vi "slow_control_2_17.vi"() -> ()   [LabVIEW 2018]
uses:
  4623b864-5764-45c6-9cb2-3e18237880ca.vi
  fa57f61f-0bb9-49ac-92eb-fcb40add4dbb.vi
  <vilib>/DAQmx/read.llb/DAQmx Read (Analog 1D DBL NChan 1Samp).vi
  ffb0d1b3-ef19-4e2e-b36e-7277177ef4b3.vi
  9a1acc8a-69db-4048-9e4c-bb07d66d2422.vi
  <vilib>/DAQmx/create/channels.llb/DAQmx Create Channel (AI-Voltage-Basic).vi
  <vilib>/DAQmx/create/channels.llb/DAQmx Create Channel (AI-Current-Basic).vi
  <vilib>/DAQmx/create/channels.llb/DAQmx Create Channel (AI-Temperature-RTD).vi
  <vilib>/DAQmx/miscellaneous.llb/DAQmx Fill In Error Info.vi
  <vilib>/Utility/file.llb/Read Delimited Spreadsheet (string).vi
  <instrlib>/Lake Shore 335/Lake Shore 335.lvlib
  <instrlib>/CAEN PSM/CAEN PSM.lvlib
  <resource>/objmgr/daqmx.rc
panel:
  out "Setpoint (°C)":dbl
  out "Heater Range":i32
  out "Heater (°C)":dbl
  out "Coldhead (°C)":dbl
  out "Cycle number":i32
  out "Alarm state":bool
  out "Timestamp last \nmeasured (UPS)":timestamp
  out "Auto-clear":bool
  in  "Auto-clear data?":bool
  in  "Clear data":bool
  in  "Clear data every N cycles":dbl=1000000.0
  in  "N samples":i32=30
  out "Average Flow (SLPM)":dbl caption="Flow (SLPM)"
  out "CAEN Ch. Names":string[](array[string])
  in  "Cycles to execute":dbl=5.0 format="%#_13g"
  out "Detector Pressure":dbl
  in  "N samples":i32=20
  in  "Allows tabs on \nfront panel":T1(tab)
  in  "Anode ch.":enum16{"1", "2", "3", "4"}(ring)=enum."3"
  in  "CAEN unit selector":enum16{"CAEN 1", "CAEN 2"}(ring)
  in  "Multipliers":dbl[](array[numeric])=[1.0, 1.0, 1.0, 1.0, 1.0, 1.0, 1.0, 1.0]
  in  "Offsets\nsubtracted":dbl[](array[numeric])=[0.0, 0.0, 0.0, 0.0, 0.0, 0.0, 0.0, 0.0]
  in  "Channel Names (9207, ai8:15)":string[](array[string])=["i0", "i1", "i2", "i3", "i4", "i5", "i6", "i7"] caption="\"Other\""
  in  "Flow meter input:":u16(ring)=3 items=["v0", "v1", "v2", "v3", "v4", "v5", "v6", "v7"]
  in  "Detector pressure input:":u16(ring) items=["v0", "v1", "v2", "v3", "v4", "v5", "v6", "v7"]
  in  "Channel Names (9207, ai0:7)":string[](array[string])=["v0", "v1", "v2", "v3", "v4", "v5", "v6", "v7"] caption="\"Other\""
  in  "Multipliers":dbl[](array[numeric])=[1.0, 1.0, 1.0, 1.0, 1.0, 1.0, 1.0, 1.0]
  in  "Offsets\nsubtracted":dbl[](array[numeric])=[0.0, 0.0, 0.0, 0.0, 0.0, 0.0, 0.0, 0.0]
  in  "Voltage channels":tag[](array[tag])=["9207/ai0", "9207/ai1", "9207/ai2", "9207/ai3", "9207/ai4", "9207/ai5", "9207/ai6", "9207/ai7"]
  in  "COM-ports CAEN":refnum<visa-resource-name>[](array[refnum])
  in  "ID Query":bool
  in  "COM-port LakeShore":refnum<visa-resource-name>
  in  "PID settings":cluster{"P":dbl, "I":dbl, "D":dbl}={"P"=50.0, "I"=20.0, "D"=120.0}
  in  "Current channels":tag[](array[tag])=["9207/ai8", "9207/ai9", "9207/ai10", "9207/ai11", "9207/ai12", "9207/ai13", "9207/ai14", "9207/ai15"]
  in  "Channel Names (CAEN)":string[](array[string])=["PMT 1", "PMT 2", "Anode", "Cathode", "Top gate", "Bottom gate", "Other 1", "Other 2"]
  in  "RTD Type":i32(ring)=10071 items=["Pt3750"=12481, "Pt3851"=10071, "Pt3911"=12482, "Pt3916"=10069, "Pt3920"=10053, "Pt3928"=12483, "Custom"=10137]
  in  "Module 1 channels (slot 1)":tag[](array[tag])=["cDAQ2Mod2/ai0", "cDAQ2Mod2/ai1", "cDAQ2Mod2/ai2", "cDAQ2Mod2/ai3", "cDAQ2Mod2/ai4", "cDAQ2Mod2/ai5", "cDAQ2Mod2/ai6", "cDAQ2Mod2/ai7"]
  in  "Resistance Configuration":i32(ring)=3 items=["3-Wire"=3, "4-Wire"=4]
  in  "R (T = 0°C):":dbl=100.0 format="%_4g"
  in  "B":dbl
  in  "A":dbl
  in  "C":dbl
  in  "Module 2 channels (slot 2)":tag[](array[tag])=["cDAQ2Mod3/ai0", "cDAQ2Mod3/ai1", "cDAQ2Mod3/ai2", "cDAQ2Mod3/ai3", "cDAQ2Mod3/ai4", "cDAQ2Mod3/ai5", "cDAQ2Mod3/ai6", "cDAQ2Mod3/ai7"]
  in  "Shut off heater \nif Alarm is active":bool=TRUE
  in  "Re-save headers":bool
  in  "Resistance Configuration":i32(ring)=3 items=["3-Wire"=3, "4-Wire"=4]
  in  "Module 3 channels":tag[](array[tag])
  in  "RTD Type":i32(ring)=12481 items=["Pt3750"=12481, "Pt3851"=10071, "Pt3911"=12482, "Pt3916"=10069, "Pt3920"=10053, "Pt3928"=12483, "Custom"=10137]
  in  "R (T = 0°C)":dbl=1000.0 format="%0.1f"
  in  "Ignore Initialization Errors":bool=TRUE caption="Ignore init. errors?"
  out "Started up?":bool
  in  "9216 Timing Mode":i32(ring)=14712 items=["High Resolution"=10195, "High Speed"=14712]
  in  "9207 Timing Mode":i32(ring)=14712 items=["High Resolution"=10195, "High Speed"=14712]
  in  "9226 Timing Mode":i32(ring)=14712 items=["High Resolution"=10195, "High Speed"=14712]
  in  "Kill all channels (Trip)":bool
  in  "Scale.Range:Minimum 8":dbl
  in  "Scale.Range:Maximum 8":dbl=4000.0
  in  "Scale.Range:Minimum 7":dbl
  in  "Scale.Range:Maximum 7":dbl=4000.0
  in  "Scale.Range:Minimum 6":dbl=-3000.0
  in  "Scale.Range:Maximum 6":dbl
  in  "Scale.Range:Minimum 5":dbl
  in  "Scale.Range:Maximum 5":dbl=3000.0
  in  "Scale.Range:Minimum 4":dbl=-5000.0
  in  "Scale.Range:Maximum 4":dbl
  in  "Scale.Range:Maximum 3":dbl=4000.0
  in  "Scale.Range:Minimum 3":dbl
  in  "Scale.Range:Maximum 2":dbl=1000.0
  in  "Scale.Range:Minimum 2":dbl
  out "CAEN 1.1":dbl(knob) scale=0.0..1000.0
  out "CAEN 1.1":string
  in  "Scale.Range:Maximum":dbl=1000.0
  in  "Scale.Range:Minimum":dbl
  out "CAEN 2.3 2":string
  out "CAEN 2.2 2":string
  out "Channel Names":string[](array[string])
  out "CAEN 2.3":dbl(knob) scale=0.0..4000.0
  out "CAEN 2.2":dbl(knob) scale=0.0..4000.0
  out "CAEN 2.1":string
  out "CAEN 2.0":string
  out "CAEN 1.3":string
  out "CAEN 1.2":string
  out "CAEN 1.0":string
  out "Channel Names":string[](array[string])
  in  "Set to zero (ramp down)":bool
  out "CAEN 2.1":dbl(knob) scale=0.0..-3000.0
  out "CAEN 2.0":dbl(knob) scale=0.0..3000.0
  in  "Apply Voltage":bool
  in  "VSet (V)":dbl[](array[numeric])
  in  "IMax (uA)":sgl[](array[numeric])
  in  "VMax (V)":u16[](array[numeric])
  out "CAEN 1.3":dbl(knob) scale=0.0..-5000.0
  out "CAEN 1.2":dbl(knob) scale=0.0..4000.0
  out "CAEN 1.0":dbl(knob) scale=0.0..1000.0
  out "Vmon (V)":dbl[](array[numeric])
  out "IMon (uA)":dbl[](array[numeric])
  in  "Reset anode\nperiodically?":bool
  in  "Kill every Y minutes":i32=10
  in  "Keep off for X seconds":i32=10
  out "?":bool
  out "Killed":bool
  out "Restarted":bool
  out "Anode timers":timestamp[](array[timestamp])
  out "Seconds until \nanode autokill":dbl format="%.2g"
  out "Seconds until \nanode reset":dbl format="%.2g"
  in  "Temperature channel selector":u16(ring) items=["0"=0, "1"=1, "2"=2, "3"=3, "4"=4, "5"=5, "6"=6, "7"=7, "Average"=666]
  out "Heater power (%)":cluster{timestamp[], dbl[]}[](graph)
  out "Flow (SLPM)":cluster{timestamp[], dbl[]}[](graph)
  out "9207 (ai 0:7, Volts)":cluster{timestamp[], dbl[]}[](graph)
  out "Phase Diagram":cluster{"X":dbl, "Y":dbl}[](graph)
  out "Setup Temperature (9216 0:15, °C)":cluster{timestamp[], dbl[]}[](graph)
  out "LakeShore readings":dbl[](array[numeric])
  out "Low Temperature (9226 0:7 and LakeShore A;B, °C)":cluster{timestamp[], dbl[]}[](graph)
  in  "Reset?":bool
  out "Integrated Flow (SL)":dbl
  in  "Pause?":bool
  in  "Setpoint (°C)":dbl=-100.0 format="%.1f"
  in  "Heater range":u16(ring) items=["Off", "Low (On)", "Medium", "High"]
  out "element 2":bool
  out "element":bool
  in  "T 8":bool
  in  "T 7":bool
  out "Minimum input voltage measured":dbl
  out "NI mod 2&3 status":bool
  in  "NI mod 2&3":bool
  in  "NI mod 1":bool
  in  "CAEN 2":bool
  in  "CAEN 1":bool
  in  "LakeShore":bool
  out "Comm. status":bool
  out "LakeShore status":bool
  out "NI mod1 (P) status":bool
  out "CAEN 1 status":bool
  out "CAEN 2 status":bool
  out "Initialization status":bool
  in  "\"Sound\" alarm":bool
  in  "Sound alarm\nFrequency (Hz)":dbl=1260.0
  in  "Send status email now":bool
  out "Email error":i32
  out "source":string
  in  "Number of Bonus lines":i32=1
  out "Names (optional)":string[](array[string])
  in  "Send daily email?":bool=TRUE
  in  "Phone numbers":string[](array[string])
  out "Alarm (or test) message":string
  in  "Alarm\nMaster switch":bool
  in  "Repeat Alarm SMS\nevery N minutes":dbl=15.0
  in  "Test alarm":bool
  out "Warning":bool
  in  "UPS":bool
  in  "UPS Voltage \nLower Threshold":dbl=220.0
  out "Det. P. warning":bool
  out "Boolean 6":bool
  out "Boolean 5":bool
  out "Boolean 4":bool
  out "Boolean 3":bool
  out "Boolean 2":bool
  out "Boolean":bool
  in  "T 6":bool
  in  "T 5":bool
  in  "T 4":bool
  in  "T 3":bool
  in  "T 2":bool
  in  "T 1":bool
  in  "Detector Pressure:":bool
  in  "Overpressure threshold":dbl
  in  "Underpressure threshold":dbl
  in  "High Temp threshold":dbl format="%#_13g"
  in  "Low Temp threshold":dbl format="%#_13g"
  out "Alarm active 2":bool
  out "SMS error":string
  out "Status email preview":string
  in  "Send status email at time:":string="14:00"
  in  "Email Addresses":string[](array[string])
  in  "return address":string="xamsups@gmail.com"
  out "NI 9226":errorcluster
  in  "HV Channel status":string="Click the button to request the latest High Voltage channel status.\nView another channel with the arrows, or typing 0 through 3."
  out "CAEN 1":T2(array[cluster])
  out "CAEN 2":T2(array[cluster])
  in  "Query HV status":bool
  in  "LabVIEW error code":string="Google this"
  in  "String 7":string="A checkmark means \"No error\" and false. A red X means an error occurred"
  out "\"status\"":bool
  in  "\"source\"":string="This may show two things: the latest executed VI in the task chain, in reverse order, or: which VI produced an error, with a short description. If the error can't easily be resolved, google the code."
  out "NI 9216 x2":errorcluster
  out "CAEN 1":errorcluster
  out "CAEN 2":errorcluster
  out "Lakeshore":errorcluster
  out "NI 9207":errorcluster
  out "Temp A":dbl
  out "Temp B":dbl
  in  "Temperature Channel Selector":u16(ring) items=["0", "1", "2", "3", "4", "5", "6", "7"]
  out "Historical Large Phase Diagram":cluster{dbl[], dbl[]}[](graph)
  out "Large Phase Diagram":cluster{"X":dbl, "Y":dbl}[](graph)
  in  "Temperature Channel Selector":u16(ring) items=["0"=0, "1"=1, "2"=2, "3"=3, "4"=4, "5"=5, "6"=6, "7"=7, "Average"=666]
  out "PT1000 data":dbl[](array[numeric]) format="%0.2f"
  out "9207 (V; A) Converted":dbl[](array[numeric])
  out "9216 #1 (°C)":dbl[](array[numeric])
  out "9216 #2 (°C)":dbl[](array[numeric])
  out "Raw readouts (V, mA)":dbl[](array[numeric]) format="%0.2f"
  out "Det.P input #":i32
  out "Flow input #":i32
  out "PT100 data":dbl[](array[numeric]) format="%0.2f"
  out "Polarity signs":dbl[](array[numeric])
  out "9207 (ai 8:15, Amperes)":cluster{timestamp[], dbl[]}[](graph)
  in  "Kill voltage":bool
  in  "stop":bool
  out "Voltages":dbl[](array[numeric])
  out "Time until next cycle":dbl format="%.3g"
  in  "Time per cycle (s)":i32=2 caption="Time Target (s)"
  # "Moving Averages"
  # "CAEN settings"
  # "NI 9216 Temperature settings"
  # "NI 9207 Voltage settings"
  # "NI 9207 Current settings"
  # "If RTD type is custom,\nspecify the Callendar-\nVan Dusen parameters"
  # "Anode connected to:"
  # "Channel:"
  # "Lakeshore settings"
  # "NI 9226 Temperature settings"
  # "Miscellaneous"
  # "Gain (P) (XX.X)"
  # "Reset (I) (XX.X)"
  # "Rate (D) (X.X%)"
  # "Data"
  # "Scale:"
  # "to"
  # "to"
  # "Scale:"
  # "Time of last reset"
  # "Time of last reactivation"
  # "to"
  # "Scale:"
  # "to"
  # "Scale:"
  # "Settings"
  # "Scale:"
  # "to"
  # "Scale:"
  # "to"
  # "Scale:"
  # "to"
  # "to"
  # "Scale:"
  # "Alarm indicators and arms"
  # "Detector Thresholds"
  # "Daily status email"
  # "SMS and sound alarm"
  # "Arms\nUp = Active"
  # "Alarm arms and warning lights"
  # "Temperature channels:"
  # "Uninterruptable Power Supply"
  # "Task/error information"
  # "High Voltage channel status"
  # "Error info example"
  # "Channel"
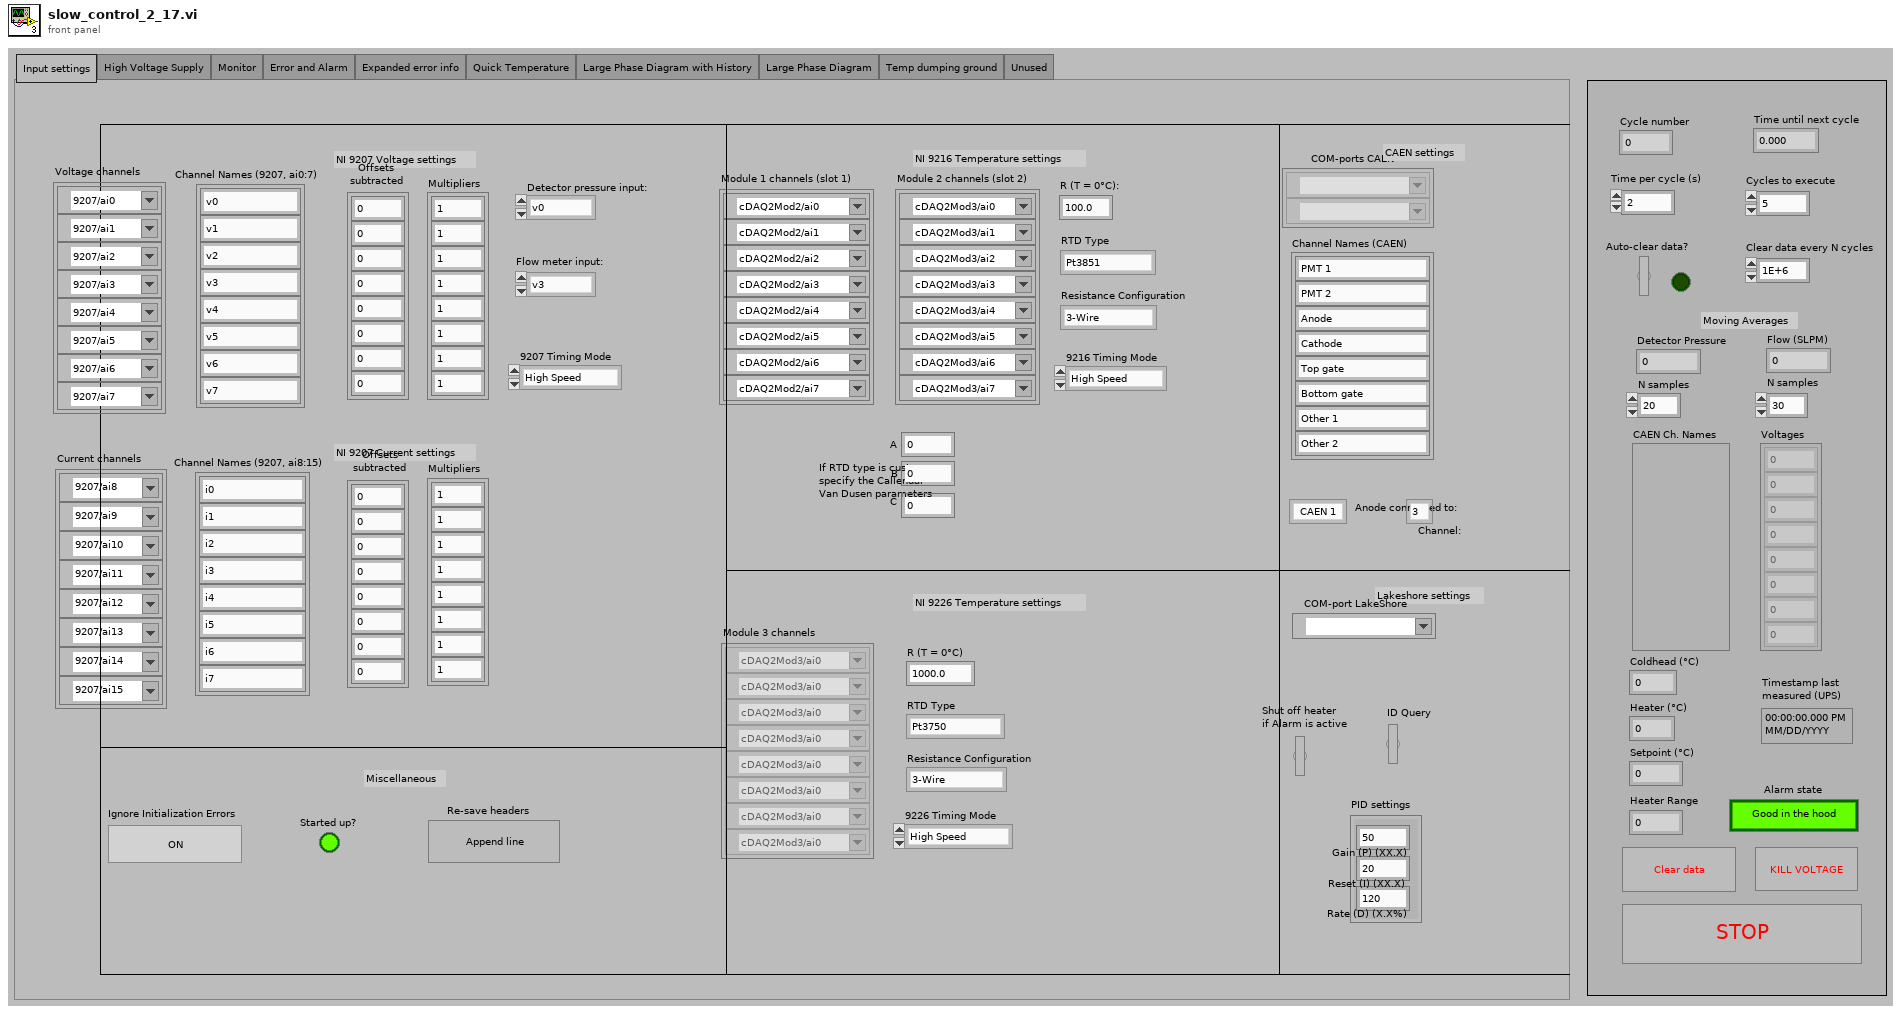
[diagram p1: front panel]
types:
  T1 = enum32{"Input settings", "High Voltage Supply", "Monitor", "Error and Alarm", "Expanded error info", "Quick Temperature", "Large Phase Diagram with History", "Large Phase Diagram", "Temp dumping ground", "Unused"}
  T2 = cluster{"ON":bool, "RUP":bool, "RDW":bool, "OVC":bool, "OVV":bool, "UNV":bool, "MAXV":bool, "TRIP":bool, "OVP":bool, "OVT":bool, "DIS":bool, "KILL":bool, "ILK":bool, "NOCAL":bool}[]
  T3 = cluster{"Baud Rate":u32, "Parity":u16, "Data Bits":u16, "Stop Bits":u16, "Flow Control":u16}
  T4 = typedef "CAEN PSM.lvlib/BoardHandle.ctl" = cluster{"VISA resource name":refnum<visa-resource-name>, "Board address":u8, "NChannels":u8}
  T5 = cluster{"task out":refnum<k21>, "error out":errorcluster}
  T6 = cluster{"VISA resource name out":refnum<visa-resource-name>, "error out":errorcluster}
  T7 = cluster{"VISA resource name":refnum<visa-resource-name>, "Board address":u8, "NChannels":u8}[]
  T8 = cluster{"VISA resource name":refnum<visa-resource-name>, "Board address":u8, "NChannels":u8}
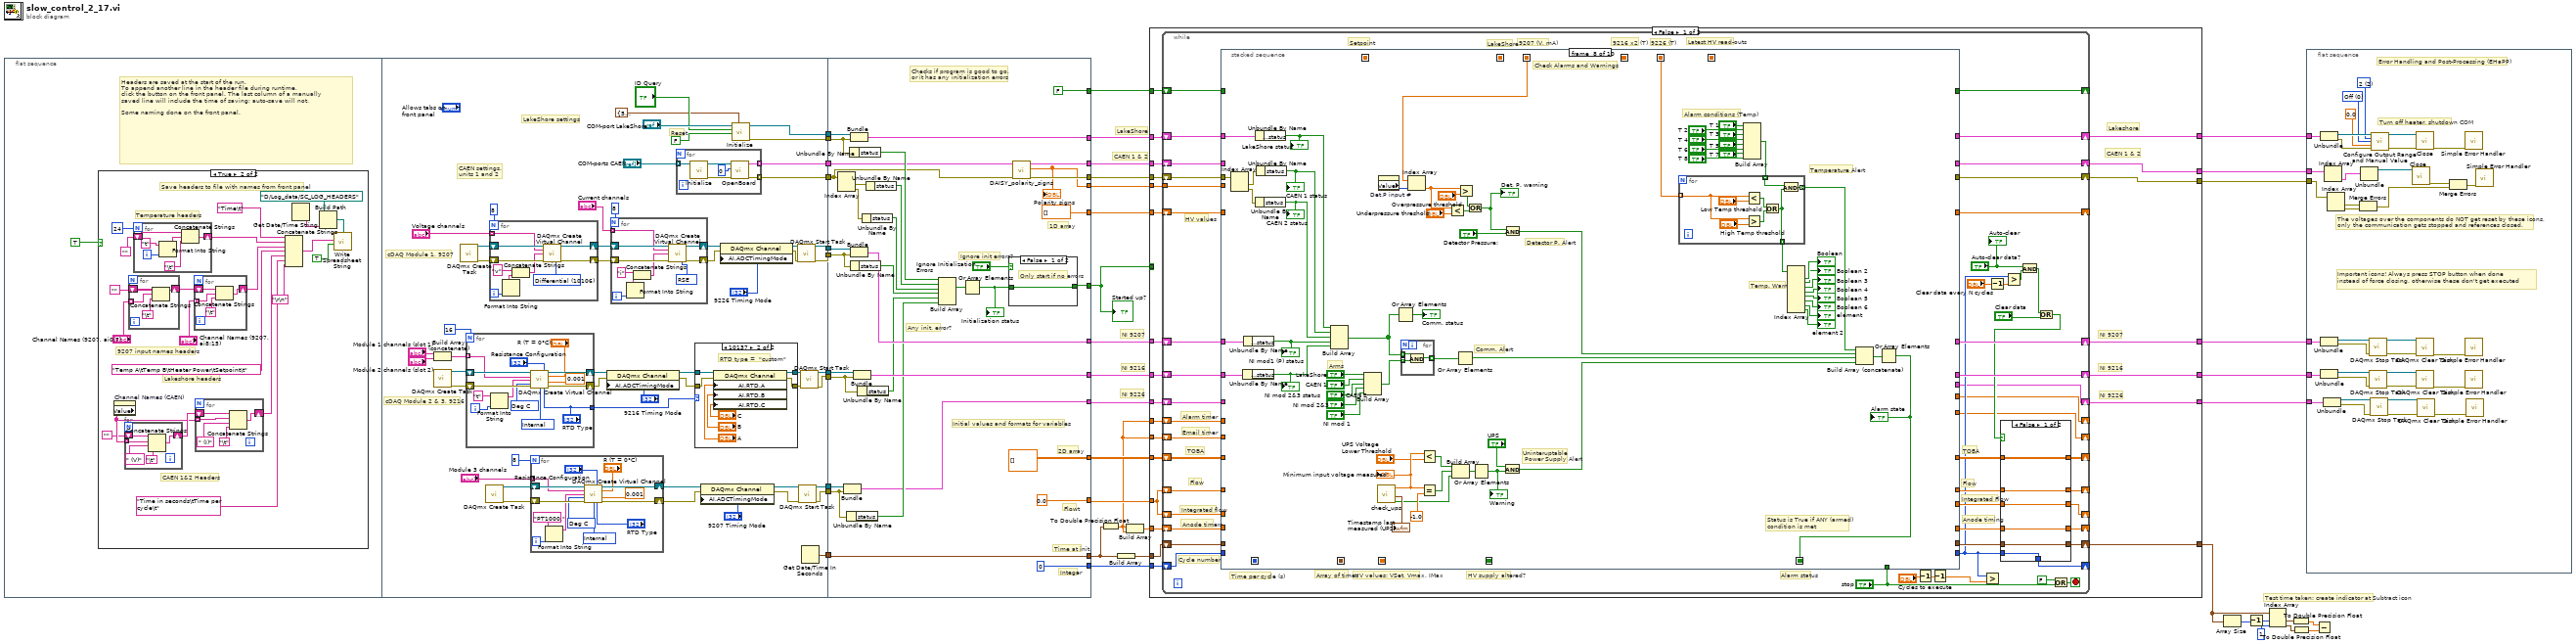
[diagram p0: block diagram]
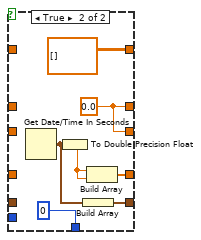
[diagram p2: hidden frame]
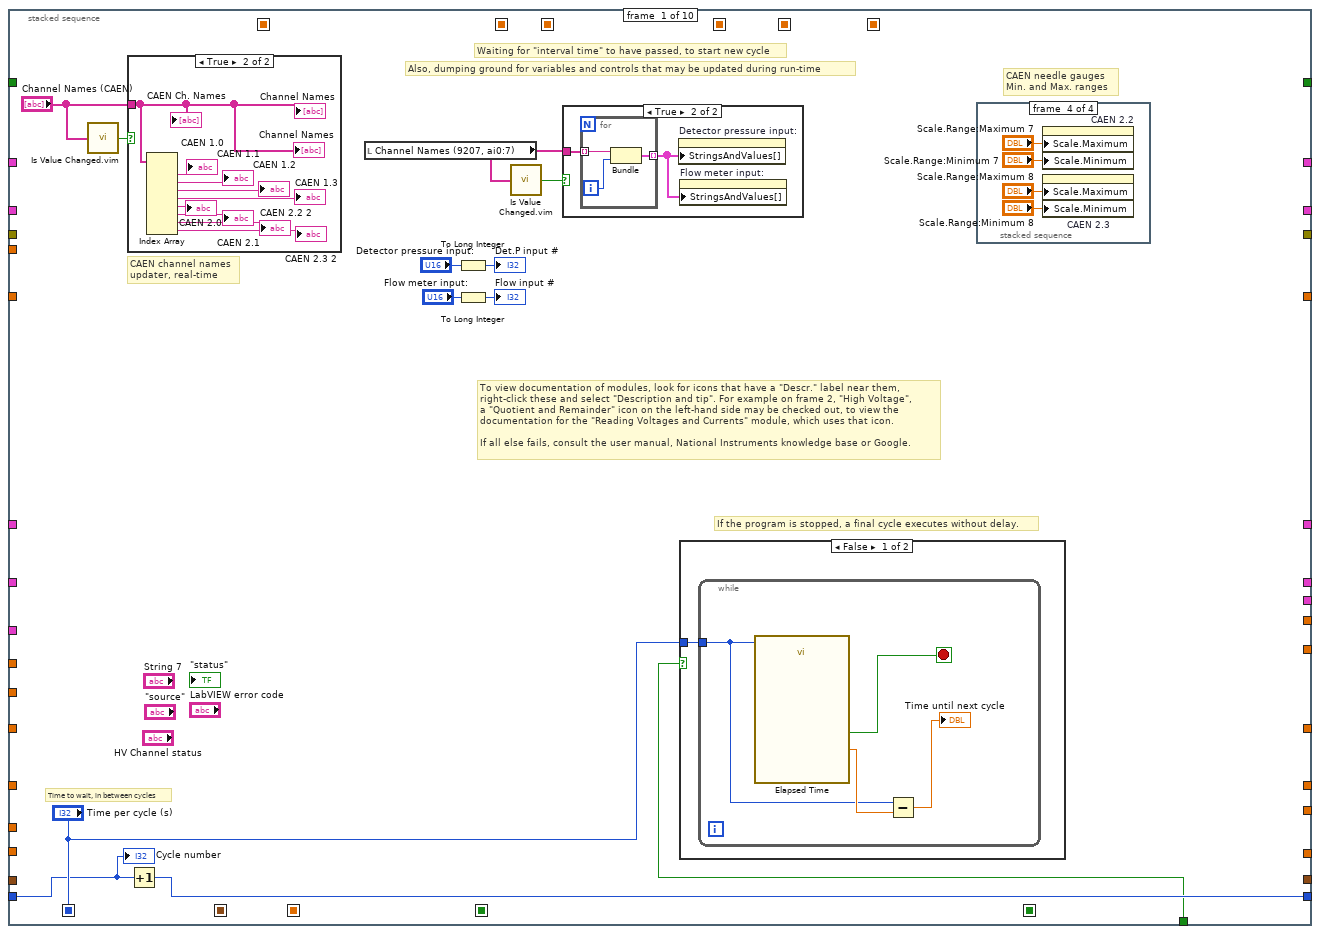
[diagram p3: hidden frame]
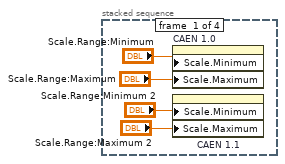
[diagram p6: hidden frame]
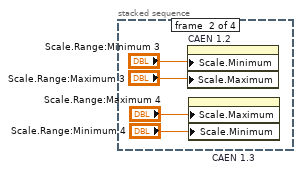
[diagram p7: hidden frame]
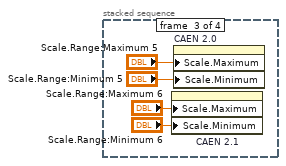
[diagram p8: hidden frame]
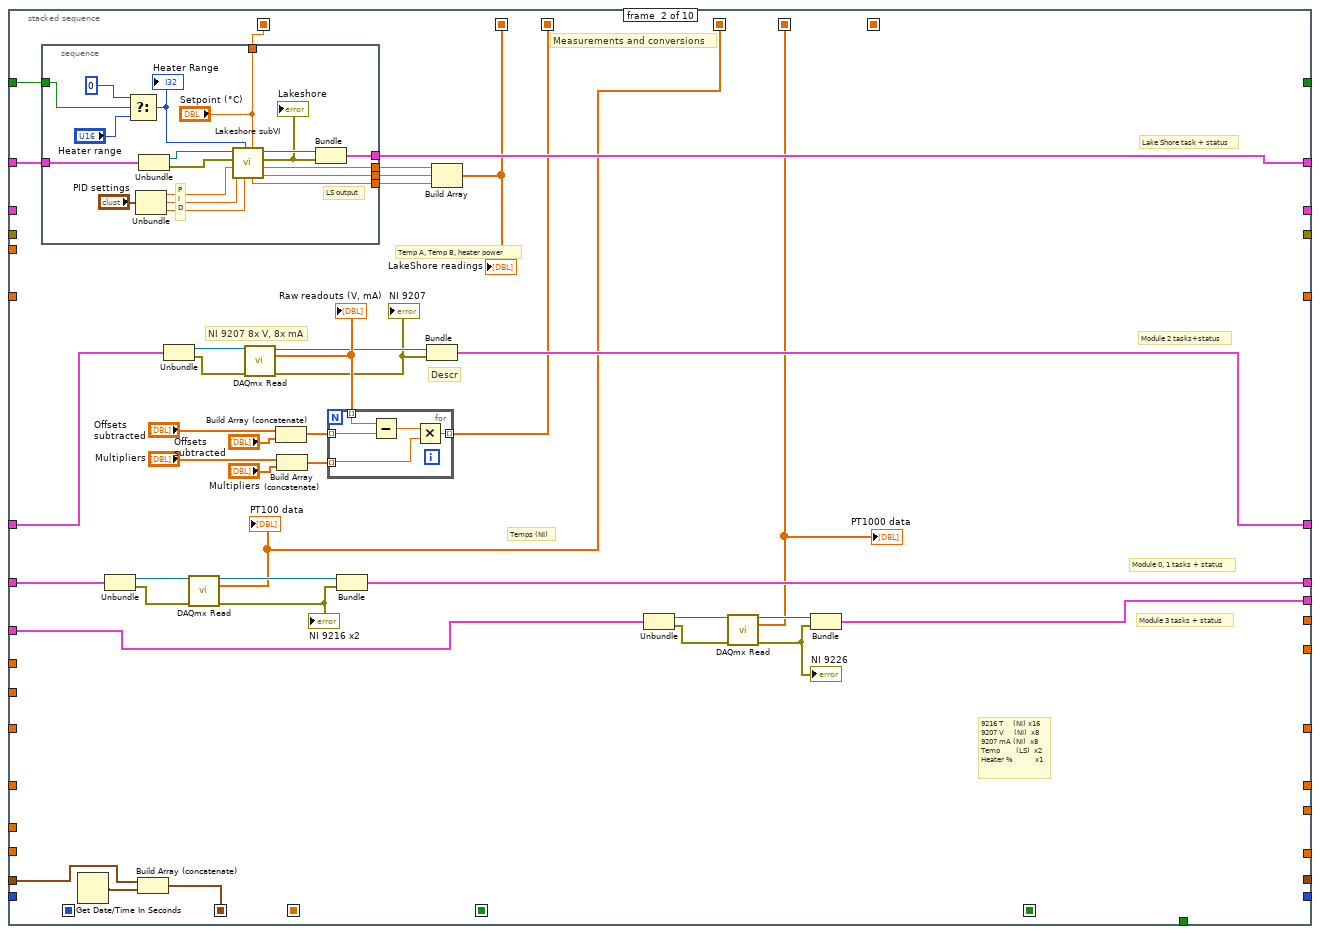
[diagram p10: hidden frame]
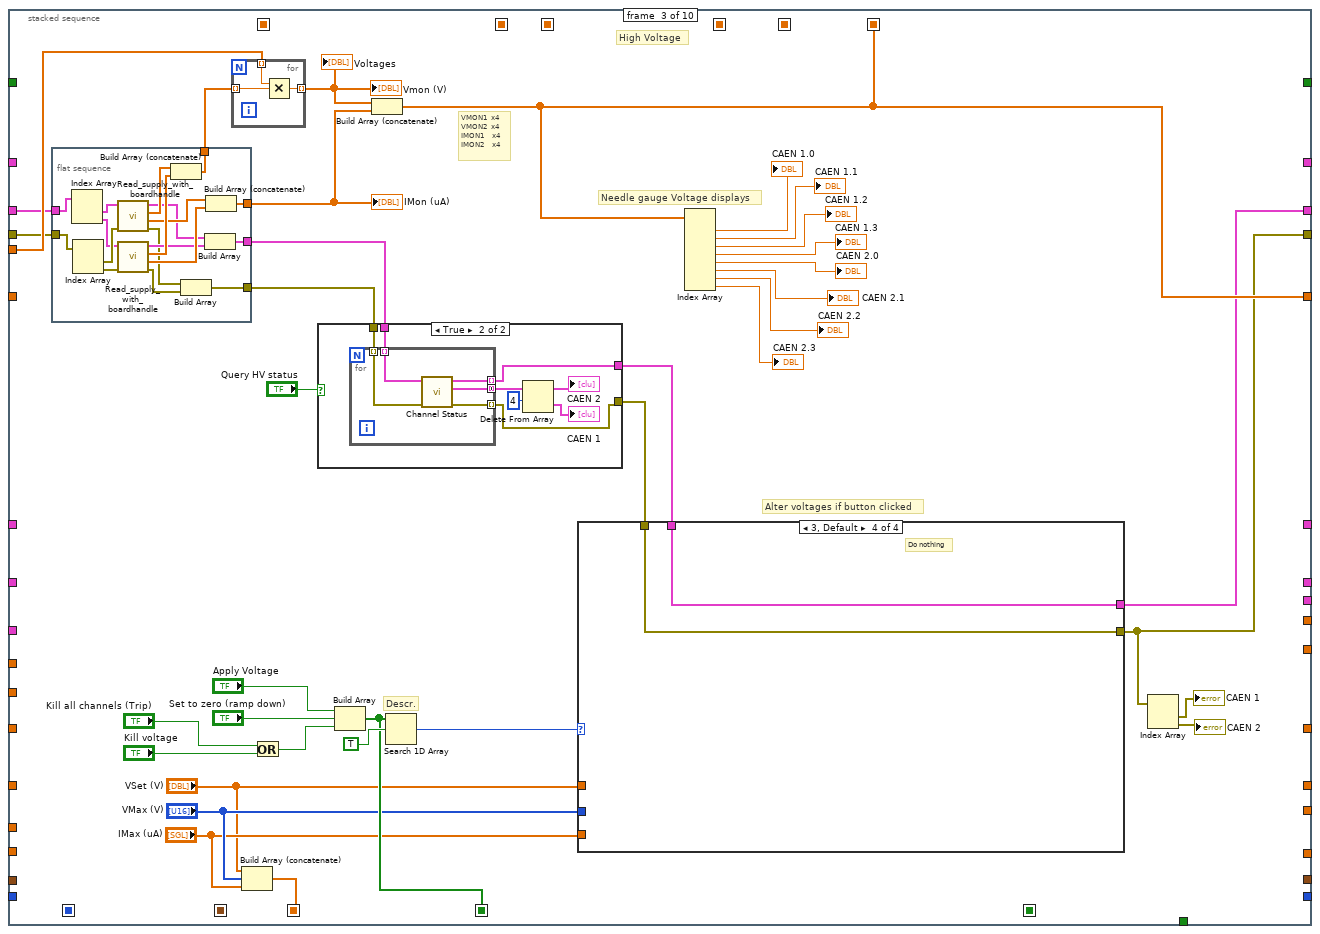
[diagram p11: hidden frame]
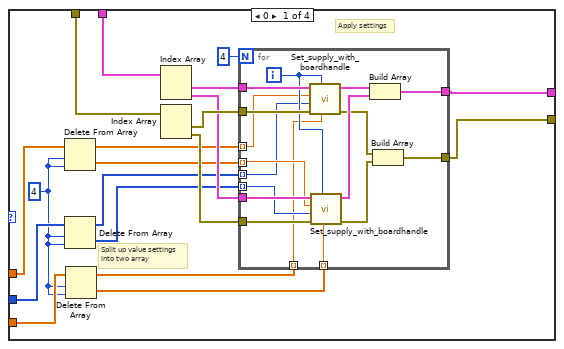
[diagram p12: hidden frame]
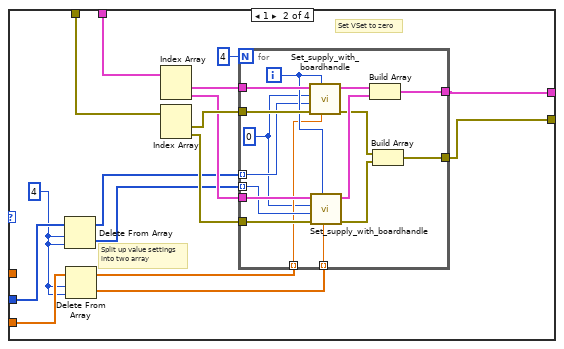
[diagram p13: hidden frame]
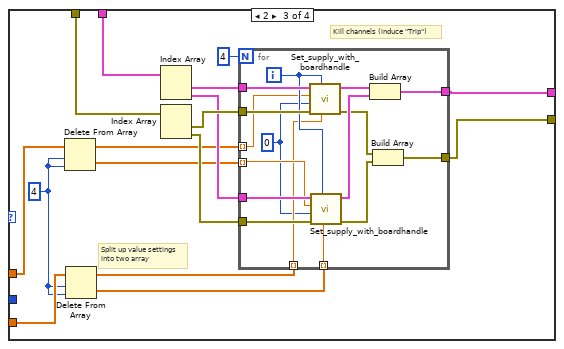
[diagram p14: hidden frame]
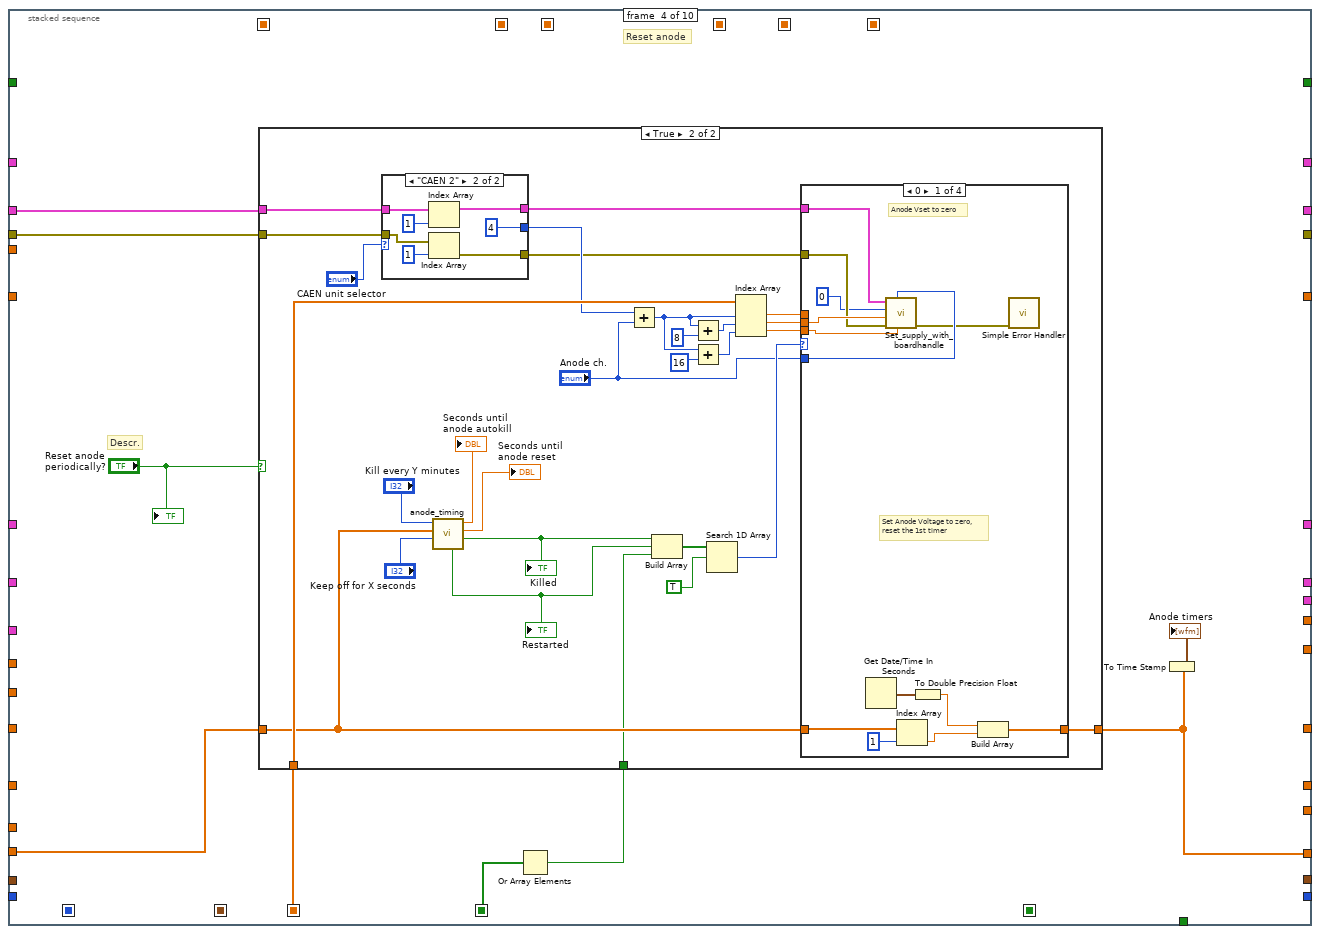
[diagram p16: hidden frame]
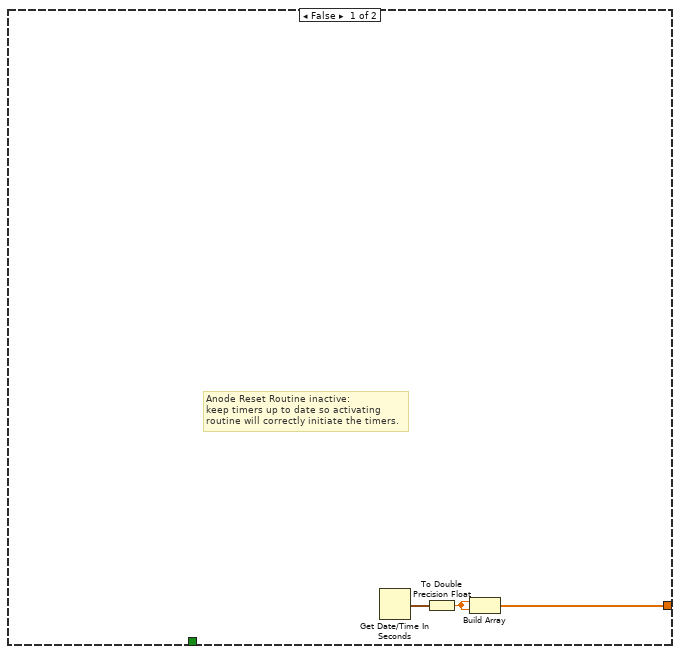
[diagram p17: hidden frame]
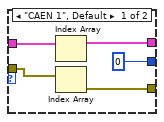
[diagram p18: hidden frame]
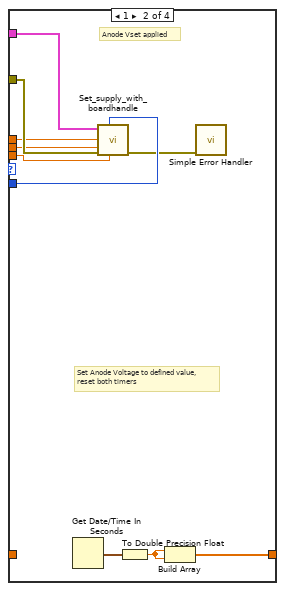
[diagram p19: hidden frame]
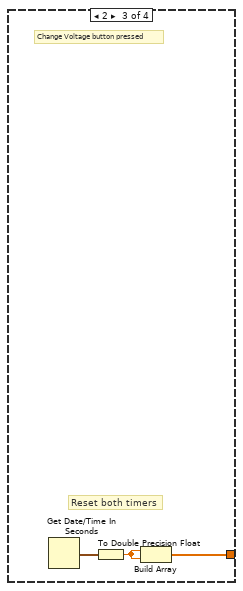
[diagram p20: hidden frame]
diagram:
  # "NI 9226"
  # "NI 9216"
  # "Test time taken: create indicator at Subtract icon"
  # "NI 9207"
  # "CAEN 1 & 2"
  # "LakeShore"
  n1 = flat-sequence {
    tunnel: [w137] -> w42
    tunnel: [w136] -> w41
    tunnel: [w135] -> w40
    tunnel: [w127] -> w39
    tunnel: [w134] -> w35
    tunnel: [w128] -> w21
    tunnel: [w122] -> w14
    tunnel: [w121] -> w13
    tunnel: [w110] -> w9
    tunnel: [w109] -> w8
    tunnel: [w106] -> w4
    tunnel: w42 -> [w235]
    tunnel: w41 -> [w234]
    tunnel: w40 -> [w206]
    tunnel: w39 -> [w227]
    tunnel: [w236] -> w27
    tunnel: [0.0] -> w26
    tunnel: [dbl[] []] -> w38
    tunnel: [dbl[][] []] -> w15
    tunnel: [0] -> w37
    tunnel: [w233] -> w36
    tunnel: [w232] -> w25
    tunnel: w35 -> [w232]
    tunnel: [FALSE] -> w22
    tunnel: w21 -> [w228]
    tunnel: [w226] -> w20
    tunnel: w14 -> [w219]
    tunnel: w13 -> [w218]
    tunnel: [w217] -> w12
    tunnel: w9 -> [w214]
    tunnel: w8 -> [w213]
    tunnel: [w211] -> w7
    tunnel: [w204] -> w5
    tunnel: w4 -> [w208]
    tunnel: [w207] -> w3
    tunnel: [w205] -> w2
    frame #0 {
      # "Headers are saved at the start of the run.\nTo append another line in the header file during runtime,\nclick the button on the front panel. The last column of a manually\nsaved line will include the time of saving; auto-save will not.\n\nSome naming done on the front panel."
      n2 = case shown="True" TRUE {
        frame False {
        }
        frame True {
          # "CAEN 1&2 Headers"
          # "Lakeshore headers"
          # "9207 input names headers"
          # "Temperature headers"
          # "Save headers to file with names from front panel"
          n3 = property on="Channel Names (CAEN)" class="Arr (strict)"() -> ("Value"=w49:string[])  [unwired: 2 in, 2 out]
          n4 = for {
            tunnel: w49 -> [w73] mode=indexing
            shift-right: [w71] -> w50
            shift-left: "" -> [w70]
            n5 = Concatenate Strings(w70, w73, " (V)", "\t") -> (w71:string)
          }
          n6 = for {
            shift-right: [w81] -> w53
            shift-left: "" -> [w82]
            tunnel: "Channel Names (9207, ai0:7)" -> [w79] mode=indexing
            n7 = Concatenate Strings(w82, w79, "\t") -> (w81:string)
          }
          n8 = for {
            N: 24 -> [_]
            shift-right: [w83] -> w56
            shift-left: "" -> [w84]
            i -> [w88]
            n9 = Format Into String(initial string="t", w88) -> (resulting string=w86:string)  [unwired: 2 in, 1 out]
            n10 = Concatenate Strings(w84, w86, "\t") -> (w83:string)
          }
          n11 = for {
            shift-right: [w76] -> w52
            shift-left: w53 -> [w78]
            tunnel: "Channel Names (9207, ai8:15)" -> [w75] mode=indexing
            n12 = Concatenate Strings(w78, w75, "\t") -> (w76:string)
          }
          n13 = for {
            shift-right: [w66] -> w48
            shift-left: w50 -> [w67]
            tunnel: w49 -> [w65] mode=indexing
            n14 = Concatenate Strings(w67, w65, " (I)", "\t") -> (w66:string)
          }
          n15 = Concatenate Strings("Time\t", w56, w52, "Temp A\tTemp B\tHeater Power\tSetpoint\t", w48, "Time in seconds\tTime per cycle\t", "\r\n") -> (w55:string)
          n16 = Get Date/Time String() -> (date string=w59:string)  [unwired: 3 in, 1 out]
          n17 = Build Path(base path=path "D:/Log_data/SC_LOG_HEADERS" ("file path (dialog if empty)"), name or relative path=w59) -> (appended path=w60:path)
          n18 = call <vilib>:"Write Spreadsheet String.vi"("append to file? (new file:F)"=TRUE, "spreadsheet string"=w55, "file path (dialog if empty)"=w60) -> ()  [unwired: 7 in, 2 out]
        }
      }
    }
    frame #1 {
      # "cDAQ Module 2 & 3, 9216"
      # "cDAQ Module 1, 9207"
      # "CAEN settings,\nunits 1 and 2"
      # "Reset"
      # "LakeShore settings"
      n19 = call <vilib>:"DAQmx Create Task.vi"() -> ("task out"=w107:refnum<k21>, "error out"=w123:errorcluster)  [unwired: 14 in]
      n20 = Build Array (concatenate)("Module 1 channels (slot 1)", "Module 2 channels (slot 2)") -> (w118:tag[])
      n21 = call <vilib>:"DAQmx Create Task.vi"() -> ("task out"=w132:refnum<k21>, "error out"=w131:errorcluster)  [unwired: 14 in]
      n22 = for {
        N: 16 -> [_]
        shift-right: [w180] -> w99
        shift-left: w107 -> [w183]
        shift-right: [w181] -> w97
        shift-left: w123 -> [w182]
        tunnel: w118 -> [w179] mode=indexing
        tunnel: ["RTD Type"] -> w115
        i -> [w177]
        w175 = 10200 items=["Internal"=10200, "External"=10167, "None"=10230] ("Current Excitation Source")
        w174 = 10143 items=["Deg C"=10143, "Deg F"=10144, "Kelvins"=10325, "Deg R"=10145, "From Custom Scale"=10065] ("units")
        n23 = Format Into String(initial string="t", w177) -> (resulting string=w176:string)  [unwired: 2 in, 1 out]
        n24 = call-poly <vilib>:"DAQmx Create Virtual Channel.vi"("task in"=w183, "resistance configuration"="Resistance Configuration", "physical channels"=w179, "r0"="R (T = 0°C):", "name to assign"=w176, "units"=w174, "current excitation value"=0.001, "error in"=w182, "current excitation source"=w175, "rtd type"="RTD Type") -> ("task out"=w180:refnum<k21>, "error out"=w181:errorcluster)  [unwired: 4 in]
      }
      n25 = call <vilib>:"DAQmx Create Task.vi"() -> ("task out"=w113:refnum<k21>, "error out"=w112:errorcluster)  [unwired: 14 in]
      n26 = for {
        N: 8 -> [_]
        shift-right: [w199] -> w105
        shift-left: w132 -> [w198]
        shift-right: [w200] -> w129
        shift-left: w131 -> [w196]
        tunnel: "Voltage channels" -> [w197] mode=indexing
        i -> [w202]
        w194 = 10106 items=["Default"=-1, "RSE"=10083, "NRSE"=10078, "Differential"=10106, "Pseudodifferential"=12529] ("input terminal configuration")
        n27 = Format Into String(w202) -> (resulting string=w201:string)  [unwired: 3 in, 1 out]
        n28 = Concatenate Strings("v" ("string"), w201) -> (w195:string)
        n29 = call-poly <vilib>:"DAQmx Create Virtual Channel.vi"("task in"=w198, "input terminal configuration"=w194, "physical channels"=w197, "name to assign"=w195, "error in"=w196) -> ("task out"=w199:refnum<k21>, "error out"=w200:errorcluster)  [unwired: 9 in]
      }
      n30 = for {
        N: 8 -> [_]
        shift-right: [w158] -> w104
        shift-left: w113 -> [w157]
        shift-right: [w159] -> w103
        shift-left: w112 -> [w160]
        tunnel: "Module 3 channels" -> [w155] mode=indexing
        i -> [w153]
        w149 = 10200 items=["Internal"=10200, "External"=10167, "None"=10230] ("current excitation source")
        w151 = 10143 items=["Deg C"=10143, "Deg F"=10144, "Kelvins"=10325, "Deg R"=10145, "From Custom Scale"=10065] ("units")
        n31 = Format Into String(initial string="PT1000.", w153) -> (resulting string=w152:string)  [unwired: 2 in, 1 out]
        n32 = call-poly <vilib>:"DAQmx Create Virtual Channel.vi"("task in"=w157, "resistance configuration"="Resistance Configuration", "physical channels"=w155, "r0"="R (T = 0°C)", "name to assign"=w152, "units"=w151, "current excitation value"=0.001, "error in"=w160, "current excitation source"=w149, "rtd type"="RTD Type") -> ("task out"=w158:refnum<k21>, "error out"=w159:errorcluster)  [unwired: 4 in]
      }
      n33 = property class="DAQmx Channel"(reference=w99, error in=w97, "AI.ADCTimingMode"="9216 Timing Mode") -> (reference out=w98:refnum<k21>, error out=w96:errorcluster)
      n34 = for {
        N: 8 -> [_]
        shift-right: [w185] -> w94
        shift-left: w105 -> [w192]
        shift-right: [w184] -> w91
        shift-left: w129 -> [w191]
        tunnel: "Current channels" -> [w190] mode=indexing
        i -> [w189]
        w193 = 10083 items=["default"=-1, "RSE"=10083, "NRSE"=10078, "Differential"=10106, "Pseudodifferential"=12529] ("input terminal configuration")
        n35 = Format Into String(w189) -> (resulting string=w187:string)  [unwired: 3 in, 1 out]
        n36 = Concatenate Strings("i", w187) -> (w186:string)
        n37 = call-poly <vilib>:"DAQmx Create Virtual Channel.vi"("task in"=w192, "input terminal configuration"=w193, "physical channels"=w190, "name to assign"=w186, "error in"=w191) -> ("task out"=w185:refnum<k21>, "error out"=w184:errorcluster)  [unwired: 9 in]
      }
      n38 = for {
        tunnel: [w145] -> w106 mode=indexing
        tunnel: [w146] -> w135 mode=indexing
        tunnel: "COM-ports CAEN" -> [w142] mode=indexing
        n39 = call <instrlib>:"Initialize.vi"("VISA resource name"=w142) -> ("error out"=w143:errorcluster, "VISA resource name out"=w144:refnum<visa-resource-name>)  [unwired: 9 in]
        n40 = call <instrlib>:"OpenBoard.vi"("error in (no error)"=w143, "Board Address"=u8 0, "VISA resource name"=w144) -> ("error out"=w146:errorcluster, "BoardHandle"=w145:T4)  [unwired: 7 in]
      }
      n41 = case shown="10137" w115 {
        tunnel: w98 -> [w162 w166]
        tunnel: w96 -> [w161 w165]
        tunnel: [w162 w164] -> w117
        tunnel: [w161 w163] -> w116
        frame 0, Default {
          # "Don't need to specify the A, B, C\nvalues if RTD type is not \"custom\""
        }
        frame 10137 {
          # "RTD type =  \"custom\""
          n42 = property class="DAQmx Channel"(reference=w166, error in=w165, "AI.RTD.A"="A", "AI.RTD.B"="B", "AI.RTD.C"="C") -> (reference out=w164:refnum<k21>, error out=w163:errorcluster)
        }
      }
      n43 = property class="DAQmx Channel"(reference=w104, error in=w103, "AI.ADCTimingMode"="9207 Timing Mode") -> (reference out=w101:refnum<k21>, error out=w100:errorcluster)
      n44 = property class="DAQmx Channel"(reference=w94, error in=w91, "AI.ADCTimingMode"="9226 Timing Mode") -> (reference out=w93:refnum<k21>, error out=w92:errorcluster)
      n45 = call <instrlib>:"Initialize.vi"("Serial Configuration"=T3 {"Baud Rate"=57600, "Parity"=1, "Data Bits"=7, "Stop Bits"=10, "Flow Control"=0}, "Reset (True)"=FALSE ("Reset (LakeShore)"), "ID Query (True)"="ID Query", "VISA resource name"="COM-port LakeShore") -> ("error out"=w136:errorcluster, "VISA resource name out"=w137:refnum<visa-resource-name>)  [unwired: 6 in]
      n46 = call <vilib>:"DAQmx Start Task.vi"("task/channels in"=w93, "error in"=w92) -> ("task out"=w128:refnum<k21>, "error out"=w127:errorcluster)  [unwired: 12 in]
      n47 = call <vilib>:"DAQmx Start Task.vi"("task/channels in"=w101, "error in"=w100) -> ("task out"=w110:refnum<k21>, "error out"=w109:errorcluster)  [unwired: 12 in]
      n48 = call <vilib>:"DAQmx Start Task.vi"("task/channels in"=w117, "error in"=w116) -> ("task out"=w122:refnum<k21>, "error out"=w121:errorcluster)  [unwired: 12 in]
      n49 = Get Date/Time In Seconds() -> (seconds since 1Jan1904=w134:timestamp)
    }
    frame #2 {
      # "1D array"
      # "Initial values and formats for variables"
      # "Time at init."
      # "Integer"
      # "2D array"
      # "Flowt"
      # "Checks if program is good to go,\nor it has any initialization errors"
      # "Ignore init errors?"
      # "Any init. error?"
      n50 = Index Array(array=w206) -> (element #1=w210:errorcluster, element #2=w209:errorcluster)  [unwired: 2 in]
      n51 = Bundle("task out"=w214, "error out"=w213) -> (w211:T5)  [unwired: 1 in]
      n52 = Unbundle By Name(w213) -> ("status"=w212:bool)
      n53 = Unbundle By Name(w234) -> ("status"=w220:bool)
      n54 = Bundle("VISA resource name out"=w235, "error out"=w234) -> (w233:T6)  [unwired: 1 in]
      n55 = Unbundle By Name(w227) -> ("status"=w221:bool)
      n56 = Bundle("task out"=w228, "error out"=w227) -> (w226:T5)  [unwired: 1 in]
      n57 = Bundle("task out"=w219, "error out"=w218) -> (w217:T5)  [unwired: 1 in]
      n58 = Unbundle By Name(w218) -> ("status"=w216:bool)
      n59 = Unbundle By Name(w209) -> ("status"=w231:bool)
      n60 = Unbundle By Name(w210) -> ("status"=w237:bool)
      n61 = Build Array(w220, w237, w221, w231, w216, w212) -> (w238:bool[])
      n62 = Or Array Elements(Boolean array=w238) -> (logical OR=w215:bool)
      "Initialization status" <- w215
      n63 = case shown="False" "Ignore Initialization Errors" {
        tunnel: [w239 FALSE] -> w236
        tunnel: w215 -> [w239 _]
        frame False {
          # "Only start if no errors"
        }
        frame True {
          # "Always start program"
        }
      }
      n64 = call "DAISY_polarity_signs.vi"("Errors in"=w206, "BoardHandles"=w208) -> ("Errors out"=w205:errorcluster[], "Polarity signs"=w204:dbl[], "BoardHandles Out"=w207:T7)  [unwired: 7 in]
      "Polarity signs" <- w204
    }
  }
  n65 = To Double Precision Float(number=w25) -> (double precision float=w10:dbl)
  n66 = Build Array(w25) -> (w34:timestamp[])
  n67 = Build Array(w10, w10) -> (w24:dbl[])
  n68 = case shown="False" w27 {
    selector: w27 -> [_ w1134]
    tunnel: [_ w1134] -> _
    tunnel: w38 -> [w258 _]
    tunnel: w37 -> [w263 _]
    tunnel: w15 -> [w262 _]
    tunnel: w36 -> [w259 w1132]
    tunnel: w34 -> [w261 _]
    tunnel: [w260 timestamp[] []] -> w30
    tunnel: w26 -> [w254 _]
    tunnel: w24 -> [w257 _]
    tunnel: [w256 w1132] -> w23
    tunnel: w22 -> [w255 _]
    tunnel: w20 -> [w253 w1131]
    tunnel: [w252 w1128] -> w19
    tunnel: [w251 w1131] -> w18
    tunnel: w12 -> [w250 w1130]
    tunnel: [w249 w1130] -> w11
    tunnel: w10 -> [w248 _]
    tunnel: w10 -> [w247 _]
    tunnel: w7 -> [w246 w1129]
    tunnel: [w245 w1129] -> w6
    tunnel: w5 -> [w244 _]
    tunnel: w3 -> [w243 w1128]
    tunnel: w2 -> [w242 w1127]
    tunnel: [w241 w1127] -> w1
    frame False {
      # "NI 9226"
      # "NI 9216"
      # "NI 9207"
      # "CAEN 1 & 2"
      # "Lakeshore"
      n69 = while {
        shift-right: [w279] -> _
        shift-left: w263 -> [w315]
        shift-right: [w292] -> _
        shift-left: w262 -> [w306]
        shift-right: [w284] -> w260
        shift-left: w261 -> [w312]
        shift-right: [w307] -> w252
        shift-left: w243 -> [w301]
        shift-right: [w309] -> _
        shift-left: w258 -> [w311]
        shift-right: [w308] -> w256
        shift-left: w259 -> [w310]
        shift-right: [w288] -> _
        shift-left: w254 -> [w303]
        shift-right: [w290] -> _
        shift-left: w254 -> [w304]
        shift-right: [w286] -> _
        shift-left: w257 -> [w302]
        shift-right: [w274] -> _
        shift-left: w255 -> [w300]
        shift-right: [w298] -> w251
        shift-left: w253 -> [w299]
        shift-right: [w296] -> w249
        shift-left: w250 -> [w297]
        shift-right: [w272] -> _
        shift-left: w248 -> [w273]
        shift-right: [w269] -> _
        shift-left: w247 -> [w270]
        shift-right: [w267] -> w245
        shift-left: w246 -> [w268]
        tunnel: w244 -> [w266]
        shift-right: [w264] -> w241
        shift-left: w242 -> [w265]
        stop <- w313 stop-if-true
        # "9226 (T)"
        # "Email timer"
        # "Alarm timer"
        # "Alarm status"
        # "LakeShore"
        # "9216 x2 (T)"
        # "9207 (V, mA)"
        # "HV supply altered?"
        # "Setpoint"
        # "Anode timing"
        # "Anode timers"
        # "Integrated flow"
        # "Flow"
        # "Flow"
        # "Integrated Flow"
        # "TOBA"
        # "Array of times"
        # "Latest HV read-outs"
        # "Time per cycle (s)"
        # "Cycle number"
        # "HV values: VSet, Vmax, IMax"
        # "HV values"
        # "TOBA"
        n70 = stacked-sequence {
          seq-local: [_ _ w467 _ _ _ _ _ _ _] -> [_ _ _ w618 _ _ _ _ _ _]
          seq-local: ["Time per cycle (s)" _ _ _ _ _ _ _ _ _] -> [_ _ _ _ _ _ w829 _ _ _]
          seq-local: [_ _ w455 _ _ _ _ _ _ _] -> [_ _ _ _ _ _ w827 _ _ _]
          seq-local: [_ w411 _ _ _ _ _ _ _ _] -> [_ _ _ _ w691 w812 _ _ _ _]
          seq-local: [_ _ w463 _ _ _ _ _ _ _] -> [_ _ _ w614 _ _ _ _ _ _]
          seq-local: [_ w405 _ _ _ _ _ _ _ _] -> [_ _ _ _ _ w801 w826 _ _ _]
          seq-local: [_ w403 _ _ _ _ _ _ _ _] -> [_ _ _ _ w713 w804 w824 w940 w970 w1056]
          seq-local: [_ w376 _ _ _ _ _ _ _ _] -> [_ _ _ _ w716 w807 w831 _ _ _]
          seq-local: [_ w391 _ _ _ _ _ _ _ _] -> [_ _ _ _ w715 w806 w825 _ _ _]
          seq-local: [_ _ _ _ _ _ _ w900 _ _] -> [_ _ _ _ _ _ _ _ w972 w1057]
          seq-local: [_ w379 _ _ _ _ _ _ _ _] -> [_ _ _ _ w702 w800 w823 w898 w966 w1039]
          tunnel: [w340 _ _ _ _ _ _ _ _ _] -> w278
          tunnel: "stop" -> [w339 _ _ _ _ _ _ _ _ _]
          tunnel: w315 -> [w329 _ _ _ _ _ _ _ _ _]
          tunnel: w306 -> [_ _ _ _ w745 _ _ _ _ _]
          tunnel: [_ _ _ _ w700 _ _ _ _ _] -> w293
          tunnel: w312 -> [_ w385 _ _ _ _ _ _ _ _]
          tunnel: w301 -> [_ _ w443 w619 _ _ _ _ _ _]
          tunnel: w311 -> [_ _ _ _ _ _ _ _ _ _]
          tunnel: w310 -> [_ w413 _ _ _ _ _ w954 _ _]
          tunnel: [_ w414 _ _ _ _ _ _ _ _] -> w308
          tunnel: [_ _ w455 _ _ _ _ _ _ _] -> w309
          tunnel: [_ _ w450 _ _ _ _ _ _ _] -> w307
          tunnel: [_ _ _ _ w691 _ _ _ _ _] -> w285
          tunnel: w303 -> [_ _ _ _ _ w810 _ _ _ _]
          tunnel: w304 -> [_ _ _ _ _ w811 _ _ _ _]
          tunnel: w302 -> [_ _ _ w620 _ _ _ _ _ _]
          tunnel: [_ _ _ w615 _ _ _ _ _ _] -> w287
          tunnel: w300 -> [_ w407 _ _ _ _ _ _ _ _]
          tunnel: w299 -> [_ w406 _ _ _ _ _ w953 _ _]
          tunnel: [_ w404 _ _ _ _ _ _ _ _] -> w298
          tunnel: [_ _ _ _ _ w809 _ _ _ _] -> w289
          tunnel: [_ _ _ _ _ w808 _ _ _ _] -> w291
          tunnel: w297 -> [_ w390 _ _ _ _ _ w941 _ _]
          tunnel: [_ w386 _ _ _ _ _ _ _ _] -> w296
          tunnel: [_ _ _ _ _ _ _ _ w974 _] -> w274
          tunnel: w273 -> [_ _ _ _ _ _ _ _ w969 _]
          tunnel: [_ _ _ _ _ _ _ _ w967 _] -> w272
          tunnel: w270 -> [_ _ _ _ _ _ _ _ _ w1044]
          tunnel: [_ _ _ _ _ _ _ _ _ w1043] -> w269
          tunnel: w268 -> [_ w384 _ _ _ _ _ _ _ _]
          tunnel: [_ w380 _ _ _ _ _ _ _ _] -> w267
          tunnel: w266 -> [_ _ w457 _ _ _ _ _ _ _]
          tunnel: w265 -> [_ _ w442 w612 _ _ _ w897 _ _]
          tunnel: [_ _ w446 _ _ _ _ _ _ _] -> w264
          frame #0 {
            # "CAEN channel names\nupdater, real-time"
            # "Also, dumping ground for variables and controls that may be updated during run-time"
            # "CAEN needle gauges\nMin. and Max. ranges"
            # "To view documentation of modules, look for icons that have a \"Descr.\" label near them,\nright-click these and select \"Description and tip\". For example on frame 2, \"High Voltage\",\na \"Quotient and Remainder\" icon on the left-hand side may be checked out, to view the\ndocumentation for the \"Reading Voltages and Currents\" module, which uses that icon. \n\nIf all else fails, consult the user manual, National Instruments knowledge base or Google."
            # "Time to wait, in between cycles"
            # "If the program is stopped, a final cycle executes without delay."
            # "Waiting for \"interval time\" to have passed, to start new cycle"
            n71 = call "Is Value Changed.vim"("value"="Channel Names (CAEN)") -> ("changed or first call?"=w332:bool)
            n72 = case shown="True" w332 {
              tunnel: "Channel Names (CAEN)" -> [_ w346]
              frame False {
              }
              frame True {
                n73 = Index Array(array=w346) -> (element #1=→"CAEN 1.0":string, element #2=→"CAEN 1.1":string, element #3=→"CAEN 1.2":string, element #4=→"CAEN 1.3":string, element #5=→"CAEN 2.0":string, element #6=→"CAEN 2.1":string, element #7=→"CAEN 2.2 2":string, element #8=→"CAEN 2.3 2":string)  [unwired: 8 in]
                "CAEN Ch. Names" <- w346
                "Channel Names" <- w346
                "Channel Names" <- w346
              }
            }
            n74 = Increment(x=w329) -> (x+1=w340:i32)
            n75 = local read "Channel Names (9207, ai0:7)"() -> (w330:string[])
            n76 = To Long Integer(number="Detector pressure input:") -> (32bit integer=→"Det.P input #":i32)
            n77 = To Long Integer(number="Flow meter input:") -> (32bit integer=→"Flow input #":i32)
            n78 = call "Is Value Changed.vim"("value"=w330) -> ("changed or first call?"=w331:bool)
            n79 = case shown="True" w331 {
              tunnel: w330 -> [_ w342]
              frame False {
                # ":D"
              }
              frame True {
                n80 = for {
                  tunnel: w342 -> [w345] mode=indexing
                  tunnel: [w343] -> w341 mode=indexing
                  i -> [w344]
                  n81 = Bundle("Or give name if \"Other\""=w345, w344) -> (w343:cluster{"Or give name if \"Other\"":string, i32})  [unwired: 1 in]
                }
                n82 = property on="Detector pressure input:" class="Ring (strict)"("StringsAndValues[]"=w341) -> ()  [unwired: 2 in, 2 out]
                n83 = property on="Flow meter input:" class="Ring (strict)"("StringsAndValues[]"=w341) -> ()  [unwired: 2 in, 2 out]
              }
            }
            n84 = case shown="False" w339 {
              tunnel: "Time per cycle (s)" -> [w371 _]
              frame False {
                n85 = while {
                  tunnel: w371 -> [w373]
                  stop <- w375 stop-if-true
                  n86 = call "Elapsed Time"("Time Target (s)"=w373) -> ("Elapsed Time (s)"=w374:dbl, "Time has Elapsed"=w375:bool)  [unwired: 11 in, 6 out]
                  n87 = Subtract(x=w373, y=w374) -> (x-y=→"Time until next cycle":dbl)
                }
              }
              frame True {
              }
            }
            n88 = stacked-sequence {
              frame #0 {
                n89 = property on="CAEN 1.0" class="Knob (strict)"("Scale.Minimum"="Scale.Range:Minimum", "Scale.Maximum"="Scale.Range:Maximum") -> ()  [unwired: 2 in, 2 out]
                n90 = property on="CAEN 1.1" class="Knob (strict)"("Scale.Minimum"="Scale.Range:Minimum 2", "Scale.Maximum"="Scale.Range:Maximum 2") -> ()  [unwired: 2 in, 2 out]
              }
              frame #1 {
                n91 = property on="CAEN 1.2" class="Knob (strict)"("Scale.Minimum"="Scale.Range:Minimum 3", "Scale.Maximum"="Scale.Range:Maximum 3") -> ()  [unwired: 2 in, 2 out]
                n92 = property on="CAEN 1.3" class="Knob (strict)"("Scale.Maximum"="Scale.Range:Maximum 4", "Scale.Minimum"="Scale.Range:Minimum 4") -> ()  [unwired: 2 in, 2 out]
              }
              frame #2 {
                n93 = property on="CAEN 2.1" class="Knob (strict)"("Scale.Maximum"="Scale.Range:Maximum 6", "Scale.Minimum"="Scale.Range:Minimum 6") -> ()  [unwired: 2 in, 2 out]
                n94 = property on="CAEN 2.0" class="Knob (strict)"("Scale.Maximum"="Scale.Range:Maximum 5", "Scale.Minimum"="Scale.Range:Minimum 5") -> ()  [unwired: 2 in, 2 out]
              }
              frame #3 {
                n95 = property on="CAEN 2.2" class="Knob (strict)"("Scale.Maximum"="Scale.Range:Maximum 7", "Scale.Minimum"="Scale.Range:Minimum 7") -> ()  [unwired: 2 in, 2 out]
                n96 = property on="CAEN 2.3" class="Knob (strict)"("Scale.Maximum"="Scale.Range:Maximum 8", "Scale.Minimum"="Scale.Range:Minimum 8") -> ()  [unwired: 2 in, 2 out]
              }
            }
            "Cycle number" <- w329
          }
          frame #1 {
            # "Module 3 tasks + status"
            # "Module 0, 1 tasks + status"
            # "Lake Shore task + status"
            # "Descr"
            # "NI 9207 8x V, 8x mA"
            # "Module 2 tasks+status"
            # "Temps (NI)"
            # "9216 T     (NI) x16\n9207 V     (NI)  x8\n9207 mA (NI)  x8\nTemp        (LS)  x2\nHeater %           x1"
            # "Temp A, Temp B, heater power"
            # "Measurements and conversions"
            n97 = stacked-sequence {
              tunnel: [w424] -> w414
              tunnel: w413 -> [w423]
              tunnel: [w422] -> w410
              tunnel: [w421] -> w409
              tunnel: [w420] -> w408
              tunnel: w407 -> [w418]
              tunnel: ["Setpoint (°C)"] -> w405
              frame #0 {
                # "LS output"
                # "P\nI\nD"
                n98 = Select(t=0, s=w418, f="Heater range") -> (s? t:f=w415:i32)
                "Heater Range" <- w415
                n99 = Unbundle("PID settings") -> ("P"=w429:dbl, "I"=w428:dbl, "D"=w427:dbl)
                n100 = Unbundle(w423) -> ("VISA resource name out"=w431:refnum<visa-resource-name>, "error out"=w430:errorcluster)
                n101 = call "Lakeshore subVI.vi"("Setpoint"="Setpoint (°C)", "Rate (D) (X.X %)"=w427, "Range"=w415, "Reset (I) (XX.X)"=w428, "Gain (P) (XX.X)"=w429, "error in (no error)"=w430, "VISA resource name"=w431) -> ("Input B"=w421:dbl, "Input A"=w422:dbl, "error out"=w425:errorcluster, "VISA resource name out"=w426:refnum<visa-resource-name>, "Heater 1 (%)"=w420:dbl)
                "Lakeshore" <- w425
                n102 = Bundle("VISA resource name out"=w426, "error out"=w425) -> (w424:T6)  [unwired: 1 in]
              }
            }
            n103 = Get Date/Time In Seconds() -> (seconds since 1Jan1904=w412:timestamp)
            n104 = Unbundle(w390) -> ("task out"=w389:refnum<k21>, "error out"=w388:errorcluster)
            n105 = Build Array (concatenate)(w385, w412) -> (w411:timestamp[])
            n106 = Unbundle(w406) -> ("task out"=w395:refnum<k21>, "error out"=w394:errorcluster)
            n107 = call-poly <vilib>:"DAQmx Read.vi"("task/channels in"=w389, "error in"=w388) -> ("task out"=w378:refnum<k21>, "data"=w376:dbl[], "error out"=w387:errorcluster)  [unwired: 11 in]
            "PT100 data" <- w376
            "NI 9216 x2" <- w387
            n108 = call-poly <vilib>:"DAQmx Read.vi"("task/channels in"=w395, "error in"=w394) -> ("task out"=w393:refnum<k21>, "data"=w402:dbl[], "error out"=w392:errorcluster)  [unwired: 11 in]
            "Raw readouts (V, mA)" <- w402
            "NI 9207" <- w392
            n109 = Build Array (concatenate)("Offsets\nsubtracted", "Offsets\nsubtracted") -> (w396:dbl[])
            n110 = Build Array (concatenate)("Multipliers", "Multipliers") -> (w399:dbl[])
            n111 = for {
              tunnel: w396 -> [w437] mode=indexing
              tunnel: w402 -> [w436] mode=indexing
              tunnel: w399 -> [w434] mode=indexing
              tunnel: [w433] -> w403 mode=indexing
              n112 = Subtract(x=w436, y=w437) -> (x-y=w435:dbl)
              n113 = Multiply(x=w435, y=w434) -> (x*y=w433:dbl)
            }
            n114 = Bundle("task out"=w378, "error out"=w387) -> (w386:T5)  [unwired: 1 in]
            n115 = Bundle("task out"=w393, "error out"=w392) -> (w404:T5)  [unwired: 1 in]
            n116 = Build Array(w410, w409, w408) -> (w391:dbl[])
            "LakeShore readings" <- w391
            n117 = Unbundle(w384) -> ("task out"=w377:refnum<k21>, "error out"=w383:errorcluster)
            n118 = call-poly <vilib>:"DAQmx Read.vi"("task/channels in"=w377, "error in"=w383) -> ("task out"=w382:refnum<k21>, "data"=w379:dbl[], "error out"=w381:errorcluster)  [unwired: 11 in]
            "NI 9226" <- w381
            "PT1000 data" <- w379
            n119 = Bundle("task out"=w382, "error out"=w381) -> (w380:T5)  [unwired: 1 in]
          }
          frame #2 {
            # "Alter voltages if button clicked"
            # "Descr."
            # "VMON1  x4 \nVMON2  x4\nIMON1    x4\nIMON2    x4"
            # "Needle gauge Voltage displays"
            # "High Voltage"
            n120 = flat-sequence {
              tunnel: w443 -> [w491]
              tunnel: w442 -> [w490]
              tunnel: [w483] -> w441
              tunnel: [w480] -> w440
              tunnel: [w475] -> w438
              tunnel: [w474] -> w439
              frame #0 {
                n121 = Index Array(array=w491) -> (element #1=w489:T4, element #2=w487:T4)  [unwired: 2 in]
                n122 = Index Array(array=w490) -> (element #1=w488:errorcluster, element #2=w486:errorcluster)  [unwired: 2 in]
                n123 = call "Read_supply_with_boardhandle.vi"("error in (no error)"=w488, "BoardHandle"=w489) -> ("error out"=w477:errorcluster, "IMon values (uA)"=w482:dbl[], "VMon values (V)"=w485:dbl[], "BoardHandle out"=w479:T8)  [unwired: 6 in]
                n124 = call "Read_supply_with_boardhandle.vi"("error in (no error)"=w486, "BoardHandle"=w487) -> ("error out"=w476:errorcluster, "IMon values (uA)"=w481:dbl[], "VMon values (V)"=w484:dbl[], "BoardHandle out"=w478:T8)  [unwired: 6 in]
                n125 = Build Array (concatenate)(w485, w484) -> (w483:dbl[])
                n126 = Build Array(w477, w476) -> (w475:errorcluster[])
                n127 = Build Array(w479, w478) -> (w474:T7)
                n128 = Build Array (concatenate)(w482, w481) -> (w480:dbl[])
              }
            }
            n129 = for {
              tunnel: w441 -> [w610] mode=indexing
              tunnel: w457 -> [w611] mode=indexing
              tunnel: [w609] -> w456 mode=indexing
              n130 = Multiply(x=w611, y=w610) -> (x*y=w609:dbl)
            }
            "Voltages" <- w456
            "Vmon (V)" <- w456
            n131 = Build Array (concatenate)("VSet (V)", "VMax (V)", "IMax (uA)") -> (w467:dbl[])
            n132 = Or(x="Kill all channels (Trip)", y="Kill voltage") -> (x .or. y?=w458:bool)
            n133 = case shown="True" "Query HV status" {
              tunnel: w439 -> [w595 w603]
              tunnel: w438 -> [w594 w602]
              tunnel: [w595 w597] -> w452
              tunnel: [w594 w596] -> w451
              frame False {
              }
              frame True {
                n134 = for {
                  tunnel: w603 -> [w608] mode=indexing
                  tunnel: w602 -> [w607] mode=indexing
                  tunnel: [w606] -> w597 mode=indexing
                  tunnel: [w605] -> w596 mode=indexing
                  tunnel: [w604] -> w601 mode=concatenating
                  n135 = call <instrlib>:"Channel Status.vi"("error in (no error)"=w607, "BoardHandle"=w608) -> ("error out"=w605:errorcluster, "Channel Status Array"=w604:T2, "BoardHandle out"=w606:T4)  [unwired: 7 in]
                }
                n136 = Delete From Array(array=w601, length=4) -> (deleted portion=→"CAEN 1":T2, array with subset deleted=→"CAEN 2":T2)  [unwired: 1 in]
              }
            }
            n137 = Build Array("Apply Voltage", "Set to zero (ramp down)", w458) -> (w463:bool[])
            n138 = Build Array (concatenate)(w456, w440) -> (w455:dbl[])
            n139 = Search 1D Array(1D array=w463, element=TRUE) -> (index of element=w453:i32)  [unwired: 1 in]
            n140 = case shown="3, Default" w453 {
              tunnel: w452 -> [w510 w543 w575 w593]
              tunnel: w451 -> [w509 w542 w574 w592]
              tunnel: [w504 w537 w569 w593] -> w450
              tunnel: [w492 w528 w560 w592] -> w446
              tunnel: "VSet (V)" -> [w502 _ w567 _]
              tunnel: "VMax (V)" -> [w501 w535 _ _]
              tunnel: "IMax (uA)" -> [w500 w534 w566 _]
              frame 0 {
                w497 = 4
                # "Split up value settings\ninto two array"
                # "Apply settings"
                n141 = Delete From Array(array=w502, length=w497, index=w497) -> (deleted portion=w498:dbl[], array with subset deleted=w499:dbl[])
                n142 = Delete From Array(array=w501, length=w497, index=w497) -> (deleted portion=w495:u16[], array with subset deleted=w496:u16[])
                n143 = Delete From Array(array=w500, length=w497, index=w497) -> (deleted portion=w493:sgl[], array with subset deleted=w494:sgl[])
                n144 = Index Array(array=w510) -> (element #1=w508:T4, element #2=w506:T4)  [unwired: 2 in]
                n145 = Index Array(array=w509) -> (element #1=w507:errorcluster, element #2=w505:errorcluster)  [unwired: 2 in]
                n146 = for {
                  N: 4 -> [_]
                  tunnel: w508 -> [w527]
                  tunnel: w507 -> [w526]
                  tunnel: w506 -> [w525]
                  tunnel: w505 -> [w524]
                  tunnel: [w519] -> w504
                  tunnel: [w518] -> w492
                  tunnel: w499 -> [w516] mode=indexing
                  tunnel: w498 -> [w515] mode=indexing
                  tunnel: w496 -> [w514] mode=indexing
                  tunnel: w495 -> [w513] mode=indexing
                  tunnel: w494 -> [w511] mode=indexing
                  tunnel: w493 -> [w512] mode=indexing
                  i -> [w517]
                  n147 = call "Set_supply_with_boardhandle.vi"("Current Limit (0.00 uA)"=w511, "Channel (0)"=w517, "error in (no error)"=w526, "Voltage Max (0.0 V)"=w514, "Voltage Level (0.0 V)"=w516, "BoardHandle"=w527) -> ("error out"=w521:errorcluster, "BoardHandle out"=w522:T8)  [unwired: 4 in]
                  n148 = call "Set_supply_with_boardhandle.vi"("Current Limit (0.00 uA)"=w512, "Channel (0)"=w517, "error in (no error)"=w524, "Voltage Max (0.0 V)"=w513, "Voltage Level (0.0 V)"=w515, "BoardHandle"=w525) -> ("error out"=w520:errorcluster, "BoardHandle out"=w523:T8)  [unwired: 4 in]
                  n149 = Build Array(w522, w523) -> (w519:T7)
                  n150 = Build Array(w521, w520) -> (w518:errorcluster[])
                }
              }
              frame 1 {
                w533 = 4
                # "Split up value settings\ninto two array"
                # "Set VSet to zero"
                n151 = Delete From Array(array=w535, length=w533, index=w533) -> (deleted portion=w531:u16[], array with subset deleted=w532:u16[])
                n152 = Delete From Array(array=w534, length=w533, index=w533) -> (deleted portion=w529:sgl[], array with subset deleted=w530:sgl[])
                n153 = Index Array(array=w543) -> (element #1=w541:T4, element #2=w539:T4)  [unwired: 2 in]
                n154 = Index Array(array=w542) -> (element #1=w540:errorcluster, element #2=w538:errorcluster)  [unwired: 2 in]
                n155 = for {
                  N: 4 -> [_]
                  tunnel: w541 -> [w559]
                  tunnel: w540 -> [w558]
                  tunnel: w539 -> [w557]
                  tunnel: w538 -> [w556]
                  tunnel: [w551] -> w537
                  tunnel: [w550] -> w528
                  tunnel: w532 -> [w548] mode=indexing
                  tunnel: w531 -> [w547] mode=indexing
                  tunnel: w530 -> [w545] mode=indexing
                  tunnel: w529 -> [w546] mode=indexing
                  i -> [w549]
                  w544 = 0
                  n156 = call "Set_supply_with_boardhandle.vi"("Current Limit (0.00 uA)"=w545, "Channel (0)"=w549, "error in (no error)"=w558, "Voltage Max (0.0 V)"=w548, "Voltage Level (0.0 V)"=w544, "BoardHandle"=w559) -> ("error out"=w553:errorcluster, "BoardHandle out"=w554:T8)  [unwired: 4 in]
                  n157 = call "Set_supply_with_boardhandle.vi"("Current Limit (0.00 uA)"=w546, "Channel (0)"=w549, "error in (no error)"=w556, "Voltage Max (0.0 V)"=w547, "Voltage Level (0.0 V)"=w544, "BoardHandle"=w557) -> ("error out"=w552:errorcluster, "BoardHandle out"=w555:T8)  [unwired: 4 in]
                  n158 = Build Array(w554, w555) -> (w551:T7)
                  n159 = Build Array(w553, w552) -> (w550:errorcluster[])
                }
              }
              frame 2 {
                w563 = 4
                # "Kill channels (induce \"Trip\")"
                # "Split up value settings\ninto two array"
                n160 = Delete From Array(array=w567, length=w563, index=w563) -> (deleted portion=w564:dbl[], array with subset deleted=w565:dbl[])
                n161 = Delete From Array(array=w566, length=w563, index=w563) -> (deleted portion=w561:sgl[], array with subset deleted=w562:sgl[])
                n162 = Index Array(array=w575) -> (element #1=w573:T4, element #2=w571:T4)  [unwired: 2 in]
                n163 = Index Array(array=w574) -> (element #1=w572:errorcluster, element #2=w570:errorcluster)  [unwired: 2 in]
                n164 = for {
                  N: 4 -> [_]
                  tunnel: w573 -> [w591]
                  tunnel: w572 -> [w590]
                  tunnel: w571 -> [w589]
                  tunnel: w570 -> [w588]
                  tunnel: [w583] -> w569
                  tunnel: [w582] -> w560
                  tunnel: w565 -> [w580] mode=indexing
                  tunnel: w564 -> [w579] mode=indexing
                  tunnel: w562 -> [w577] mode=indexing
                  tunnel: w561 -> [w578] mode=indexing
                  i -> [w581]
                  w576 = 0
                  n165 = call "Set_supply_with_boardhandle.vi"("Current Limit (0.00 uA)"=w577, "Channel (0)"=w581, "error in (no error)"=w590, "Voltage Max (0.0 V)"=w576, "Voltage Level (0.0 V)"=w580, "BoardHandle"=w591) -> ("error out"=w585:errorcluster, "BoardHandle out"=w586:T8)  [unwired: 4 in]
                  n166 = call "Set_supply_with_boardhandle.vi"("Current Limit (0.00 uA)"=w578, "Channel (0)"=w581, "error in (no error)"=w588, "Voltage Max (0.0 V)"=w576, "Voltage Level (0.0 V)"=w579, "BoardHandle"=w589) -> ("error out"=w584:errorcluster, "BoardHandle out"=w587:T8)  [unwired: 4 in]
                  n167 = Build Array(w586, w587) -> (w583:T7)
                  n168 = Build Array(w585, w584) -> (w582:errorcluster[])
                }
              }
              frame 3, Default {
                # "Do nothing"
              }
            }
            n169 = Index Array(array=w455) -> (element #1=→"CAEN 1.0":dbl, element #2=→"CAEN 1.1":dbl, element #3=→"CAEN 1.2":dbl, element #4=→"CAEN 1.3":dbl, element #5=→"CAEN 2.0":dbl, element #6=→"CAEN 2.1":dbl, element #7=→"CAEN 2.2":dbl, element #8=→"CAEN 2.3":dbl)  [unwired: 8 in]
            n170 = Index Array(array=w446) -> (element #1=→"CAEN 1":errorcluster, element #2=→"CAEN 2":errorcluster)  [unwired: 2 in]
            "IMon (uA)" <- w440
          }
          frame #3 {
            # "Descr."
            # "Reset anode"
            n171 = Or Array Elements(Boolean array=w614) -> (logical OR=w613:bool)
            n172 = case shown="True" "Reset anode\nperiodically?" {
              tunnel: w620 -> [_ w629]
              tunnel: w619 -> [_ w636]
              tunnel: w618 -> [_ w641]
              tunnel: w613 -> [_ w627]
              tunnel: [w621 w628] -> w615
              tunnel: w612 -> [_ w625]
              frame False {
                # "Anode Reset Routine inactive:\nkeep timers up to date so activating\nroutine will correctly initiate the timers."
                n173 = Get Date/Time In Seconds() -> (seconds since 1Jan1904=w623:timestamp)
                n174 = To Double Precision Float(number=w623) -> (double precision float=w622:dbl)
                n175 = Build Array(w622, w622) -> (w621:dbl[])
              }
              frame True {
                n176 = case shown="\"CAEN 2\"" "CAEN unit selector" {
                  tunnel: w636 -> [w656 w662]
                  tunnel: [0 4] -> w634
                  tunnel: [w654 w660] -> w626
                  tunnel: w625 -> [w653 w658]
                  tunnel: [w652 w657] -> w624
                  frame "CAEN 1", Default {
                    n177 = Index Array(array=w656) -> (element=w654:T4)  [unwired: 1 in]
                    n178 = Index Array(array=w653) -> (element=w652:errorcluster)  [unwired: 1 in]
                  }
                  frame "CAEN 2" {
                    n179 = Index Array(array=w662, index=1) -> (element=w660:T4)
                    n180 = Index Array(array=w658, index=1) -> (element=w657:errorcluster)
                  }
                }
                n181 = call "anode_timing.vi"("Keep off for X seconds"="Keep off for X seconds", "Array of timers"=w629, "Kill every Y minutes"="Kill every Y minutes") -> ("Time to kill"=w643:bool, "Time until reset"=→"Seconds until \nanode reset":dbl, "Time until autokill"=→"Seconds until \nanode autokill":dbl, "Time to reset"=w644:bool)  [unwired: 5 in]
                "Killed" <- w643
                "Restarted" <- w644
                n182 = Add(x=w634, y="Anode ch.") -> (x+y=w632:i32)
                n183 = Build Array(w643, w644, w627) -> (w647:bool[])
                n184 = Add(x=w632, y=8) -> (x+y=w637:i32)
                n185 = Add(x=w632, y=16) -> (x+y=w638:i32)
                n186 = Search 1D Array(1D array=w647, element=TRUE) -> (index of element=w646:i32)  [unwired: 1 in]
                n187 = Index Array(array=w641, index #1=w632, index #2=w637, index #3=w638) -> (element #1=w650:dbl, element #2=w648:dbl, element #3=w649:dbl)
                n188 = case shown="0" w646 {
                  tunnel: w650 -> [_ w678 _ _]
                  tunnel: w648 -> [w670 w679 _ _]
                  tunnel: w649 -> [w669 w680 _ _]
                  tunnel: "Anode ch." -> [w666 w681 _ _]
                  tunnel: w629 -> [w672 _ _ w690]
                  tunnel: [w671 w684 w687 w690] -> w628
                  tunnel: w626 -> [w667 w682 _ _]
                  tunnel: w624 -> [w668 w683 _ _]
                  frame 0 {
                    # "Set Anode Voltage to zero,\nreset the 1st timer"
                    # "Anode Vset to zero"
                    n189 = Get Date/Time In Seconds() -> (seconds since 1Jan1904=w675:timestamp)
                    n190 = call "Set_supply_with_boardhandle.vi"("Current Limit (0.00 uA)"=w669, "Channel (0)"=w666, "error in (no error)"=w668, "Voltage Max (0.0 V)"=w670, "Voltage Level (0.0 V)"=0, "BoardHandle"=w667) -> ("error out"=w665:errorcluster)  [unwired: 4 in, 1 out]
                    n191 = Index Array(array=w672, index=1) -> (element=w673:dbl)
                    n192 = To Double Precision Float(number=w675) -> (double precision float=w674:dbl)
                    n193 = Build Array(w674, w673) -> (w671:dbl[])
                    n194 = call <vilib>:"Simple Error Handler.vi"("error in (no error)"=w665) -> ()  [unwired: 4 in, 5 out]
                  }
                  frame 1 {
                    # "Set Anode Voltage to defined value,\nreset both timers"
                    # "Anode Vset applied"
                    n195 = Get Date/Time In Seconds() -> (seconds since 1Jan1904=w686:timestamp)
                    n196 = call "Set_supply_with_boardhandle.vi"("Current Limit (0.00 uA)"=w680, "Channel (0)"=w681, "error in (no error)"=w683, "Voltage Max (0.0 V)"=w679, "Voltage Level (0.0 V)"=w678, "BoardHandle"=w682) -> ("error out"=w677:errorcluster)  [unwired: 4 in, 1 out]
                    n197 = To Double Precision Float(number=w686) -> (double precision float=w685:dbl)
                    n198 = Build Array(w685, w685) -> (w684:dbl[])
                    n199 = call <vilib>:"Simple Error Handler.vi"("error in (no error)"=w677) -> ()  [unwired: 4 in, 5 out]
                  }
                  frame 2 {
                    # "Change Voltage button pressed"
                    # "Reset both timers"
                    n200 = Get Date/Time In Seconds() -> (seconds since 1Jan1904=w689:timestamp)
                    n201 = To Double Precision Float(number=w689) -> (double precision float=w688:dbl)
                    n202 = Build Array(w688, w688) -> (w687:dbl[])
                  }
                  frame 3, Default {
                    # "Timers stay at previous value,\nso difference between those and\ncurrent time keeps incrementing"
                    # "No event"
                  }
                }
              }
            }
            n203 = To Time Stamp(1:w615) -> (0:→"Anode timers":timestamp[])
            "?" <- "Reset anode\nperiodically?"
          }
          frame #4 {
            # "Det. P"
            # "Flow"
            # "Flexibly acquire indices"
            # "Plots 9207 output vs time"
            # "Descr."
            # "Moving averages"
            # "Historic graphs: Phase, 9207 ai, Flow, Heater, Temperature"
            # "Non-historic Temperature + Det. Pressure"
            # "Updated TOBA >>>"
            # "Descr."
            # "Latest Detector Pressure"
            # "Plots individual lists of Temp. vs. t"
            # "Plots and moving averages"
            n204 = Build Array (concatenate)(w716, w702, w713, w715) -> (w744:dbl[])
            n205 = Build Array (concatenate)(w745, w744) -> (w700:dbl[][])
            n206 = Array Size(array=w713) -> (size(s)=w712:i32)
            n207 = Array Size(array=w702) -> (size(s)=w714:i32)
            n208 = Array Size(array=w716) -> (size(s)=w703:i32)
            n209 = Add(x=w703, y=w714) -> (x+y=w698:i32)
            n210 = Add(x=w698, y=w712) -> (x+y=w711:i32)
            n211 = local read "Flow input #"() -> (w722:i32)
            n212 = local read "Det.P input #"() -> (w723:i32)
            n213 = Add(x=w711, y=2 ("disabled index (col)")) -> (x+y=w709:i32)
            n214 = Equal?(x=666, y="Temperature channel selector") -> (x = y?=w738:bool)
            n215 = Index Array(array=w700, index (col)=w709) -> (element=w708:dbl[])  [unwired: 1 in]
            n216 = case shown="True" w738 {
              tunnel: w702 -> [w783 w784]
              tunnel: [w782 w785] -> w736
              tunnel: "Temperature channel selector" -> [w781 _]
              frame False {
                n217 = Index Array(array=w783, index=w781) -> (element=w782:dbl)
              }
              frame True {
                n218 = Add Array Elements(numeric array=w784) -> (sum=w786:dbl)
                n219 = Array Size(array=w784) -> (size(s)=w787:i32)
                n220 = Divide(x=w786, y=w787) -> (x/y=w785:dbl)
              }
            }
            n221 = Add(x=w723, y=w698) -> (x+y=w732:i32)
            n222 = Add(x=w698, y=w722) -> (x+y=w730:i32)
            n223 = Bundle(w691, w708) -> (w705:cluster{timestamp[], dbl[]})  [unwired: 1 in]
            n224 = Build Array(w705) -> (→"Heater power (%)":cluster{timestamp[], dbl[]}[])
            n225 = Add(x=w703, y="Temperature Channel Selector") -> (x+y=w706:i32)
            n226 = Index Array(array=w700, index (col) #1=w732, index (col) #2=w730) -> (element #1=w731:dbl[], element #2=w720:dbl[])  [unwired: 2 in]
            n227 = local read "Det.P input #"() -> (w724:i32)
            n228 = Index Array(array=w700, index (col)=w706) -> (element=w735:dbl[])  [unwired: 1 in]
            n229 = for {
              N: 8 -> [_]
              tunnel: w700 -> [w774]
              tunnel: w691 -> [w767]
              tunnel: [w771] -> w728 mode=indexing
              tunnel: [w766] -> w727 mode=indexing
              tunnel: w698 -> [w764]
              i -> [w770]
              n230 = Add(x=w764, y=8) -> (x+y=w763:i32)
              n231 = Add(x=w764, y=w770) -> (x+y=w773:i32)
              n232 = Add(x=w770, y=w763) -> (x+y=w769:i32)
              n233 = Index Array(array=w774, index (col) #1=w773, index (col) #2=w769) -> (element #1=w772:dbl[], element #2=w768:dbl[])  [unwired: 2 in]
              n234 = Bundle(w767, w772) -> (w771:cluster{timestamp[], dbl[]})  [unwired: 1 in]
              n235 = Bundle(w767, w768) -> (w766:cluster{timestamp[], dbl[]})  [unwired: 1 in]
            }
            "9207 (ai 0:7, Volts)" <- w728
            "9207 (ai 8:15, Amperes)" <- w727
            n236 = Bundle(w735, w731) -> (w749:cluster{dbl[], dbl[]})  [unwired: 1 in]
            n237 = Index Array(array=w713, index=w724) -> (element=w750:dbl)
            n238 = call "moving_avg.vi"("N samples"="N samples", "Array"=w731) -> ("Numeric"=→"Detector Pressure":dbl)  [unwired: 9 in]
            n239 = call "moving_avg.vi"("N samples"="N samples", "Array"=w720) -> ("Numeric"=→"Average Flow (SLPM)":dbl)  [unwired: 9 in]
            n240 = Bundle(w691, w720) -> (w747:cluster{timestamp[], dbl[]})  [unwired: 1 in]
            n241 = Build Array(w749) -> (→"Historical Large Phase Diagram":cluster{dbl[], dbl[]}[])
            n242 = Bundle("Waveform"=w736, w750) -> (w754:cluster{"Waveform":dbl, dbl})  [unwired: 1 in]
            n243 = Build Array(w747) -> (→"Flow (SLPM)":cluster{timestamp[], dbl[]}[])
            n244 = Build Array(w754) -> (→"Phase Diagram":cluster{"Waveform":dbl, dbl}[])
            n245 = for {
              N: w703 -> [_]
              tunnel: w691 -> [w799]
              tunnel: [w798] -> w755 mode=indexing
              tunnel: w700 -> [w797]
              i -> [w795]
              n246 = Index Array(array=w797, index (col)=w795) -> (element=w796:dbl[])  [unwired: 1 in]
              n247 = Bundle(w799, w796) -> (w798:cluster{timestamp[], dbl[]})  [unwired: 1 in]
            }
            "Setup Temperature (9216 0:15, °C)" <- w755
            n248 = Increment(x=w698) -> (x+1=w699:i32)
            n249 = Array Size(array=w702) -> (size(s)=w701:i32)
            n250 = Equal?(x=666, y="Temperature Channel Selector") -> (x = y?=w740:bool)
            n251 = Index Array(array=w700, index (col) #1=w698, index (col) #2=w699) -> (element #1=w697:dbl[], element #2=w696:dbl[])  [unwired: 2 in]
            n252 = local read "Channel Names (9207, ai0:7)"() -> (w725:string[])
            n253 = local read "Channel Names (9207, ai8:15)"() -> (w726:string[])
            n254 = case shown="False" w740 {
              tunnel: w702 -> [w790 w791]
              tunnel: [w789 w792] -> w743
              tunnel: "Temperature Channel Selector" -> [w788 _]
              frame False {
                n255 = Index Array(array=w790, index=w788) -> (element=w789:dbl)
              }
              frame True {
                n256 = Add Array Elements(numeric array=w791) -> (sum=w793:dbl)
                n257 = Array Size(array=w791) -> (size(s)=w794:i32)
                n258 = Divide(x=w793, y=w794) -> (x/y=w792:dbl)
              }
            }
            n259 = for {
              N: w701 -> [_]
              tunnel: w691 -> [w762]
              tunnel: [w761] -> w695 mode=indexing
              tunnel: w700 -> [w760]
              tunnel: w703 -> [w756]
              i -> [w757]
              n260 = Add(x=w756, y=w757) -> (x+y=w758:i32)
              n261 = Index Array(array=w760, index (col)=w758) -> (element=w759:dbl[])  [unwired: 1 in]
              n262 = Bundle(w762, w759) -> (w761:cluster{timestamp[], dbl[]})  [unwired: 1 in]
            }
            n263 = Bundle(w691, w697) -> (w694:cluster{timestamp[], dbl[]})  [unwired: 1 in]
            n264 = Bundle(w691, w696) -> (w693:cluster{timestamp[], dbl[]})  [unwired: 1 in]
            n265 = call "Is Value Changed.vim"("value"=w726) -> ("changed or first call?"=w733:bool)
            n266 = call "Is Value Changed.vim"("value"=w725) -> ("changed or first call?"=w734:bool)
            n267 = case shown="True" w733 {
              tunnel: w726 -> [_ w775]
              frame False {
              }
              frame True {
                n268 = for {
                  tunnel: w775 -> [w776] mode=indexing
                  i -> [w777]
                  n269 = property on="9207 (ai 8:15, Amperes)" class="XYGraph (strict)"("Active Plot"=w777, "Plot.Plot Name"=w776) -> ()  [unwired: 2 in, 2 out]
                }
              }
            }
            n270 = case shown="True" w734 {
              tunnel: w725 -> [_ w778]
              frame False {
              }
              frame True {
                n271 = for {
                  tunnel: w778 -> [w779] mode=indexing
                  i -> [w780]
                  n272 = property on="9207 (ai 0:7, Volts)" class="XYGraph (strict)"("Active Plot"=w780, "Plot.Plot Name"=w779) -> ()  [unwired: 2 in, 2 out]
                }
              }
            }
            n273 = Bundle("Waveform"=w743, w750) -> (w752:cluster{"Waveform":dbl, dbl})  [unwired: 1 in]
            n274 = Build Array (concatenate)(w695, w694, w693) -> (→"Low Temperature (9226 0:7 and LakeShore A;B, °C)":cluster{timestamp[], dbl[]}[])
            n275 = Build Array(w752) -> (→"Large Phase Diagram":cluster{"Waveform":dbl, dbl}[])
          }
          frame #5 {
            # "Temperatures x8\nTo indicators on schematic\ninside detector"
            # "Temp A, Temp B, Heater%"
            # "Temperatures x16\nTo indicators on the physical schematic"
            # "Individual latest 9207 readings.\nIndicators go here. Array is 1x16,\nitems have been converted using\nthe offsets and multipliers"
            # "Displays"
            n276 = local read "Flow input #"() -> (w805:i32)
            n277 = case shown="False" "Reset?" {
              tunnel: [w817 0.0] -> w813
              tunnel: w810 -> [w817 _]
              frame False {
              }
              frame True {
              }
            }
            n278 = Index Array(array=w804) -> ()  [unwired: 16 in, 16 out]
            n279 = Index Array(array=w804, index=w805) -> (element=w808:dbl)
            n280 = call "Average_flow_x_time.vi"("Array of timestamps"=w812, "Previous Flow"=w811, "Latest Flow"=w808) -> ("Volume (SL)"=w814:dbl)  [unwired: 8 in]
            n281 = case shown="False" "Pause?" {
              tunnel: w813 -> [w821 w822]
              tunnel: w814 -> [w820 _]
              tunnel: [w819 w822] -> w809
              frame False {
                n282 = Add(x=w820, y=w821) -> (x+y=w819:dbl)
              }
              frame True {
              }
            }
            "Integrated Flow (SL)" <- w809
            n283 = Index Array(array=w806) -> (element #1=→"Coldhead (°C)" →"Temp A":dbl, element #2=→"Heater (°C)" →"Temp B":dbl)  [unwired: 3 in, 1 out]
            n284 = Index Array(array=w807) -> ()  [unwired: 16 in, 16 out]
            n285 = Index Array(array=w800) -> ()  [unwired: 8 in, 8 out]
            "9207 (V; A) Converted" <- w804
            "9216 #1 (°C)" <- w807
            "9216 #2 (°C)" <- w807
            "Setpoint (°C)" <- w801
          }
          frame #6 {
            # "The same order applies to the headers resaved,\nbut with an additional line, stating the date/time"
            # "-----------DATA SAVED----------\nHuman-readable timestamp  ;\nTemperatures (16),  2xNI 9216;\nTemperatures (8),        NI 9226;\nVolts, Amps  (8 x2),     NI 9207;\nTemperature (2),    Lakeshore;\nHeater power (1),  Lakeshore;\nSetpoint (1),           Lakeshore;\nHV readouts (16)          CAEN ;\nCurrent time (s)                ---   ;\nCycle time (s)                    ---   ;"
            # "Saving data"
            n286 = Get Date/Time In Seconds() -> (seconds since 1Jan1904=w845:timestamp)
            n287 = To Double Precision Float(number=w845) -> (double precision float=w828:dbl)
            n288 = Build Array (concatenate)(w831, w823, w824, w825, w826, w827, w828, w829) -> (w844:dbl[])
            n289 = Array Size(array=w831) -> (size(s)=w832:i32)
            n290 = Array Size(array=w823) -> (size(s)=w833:i32)
            n291 = Add(x=w832, y=w833) -> (x+y=w830:i32)
            n292 = Get Date/Time String() -> (date string=w838:string)  [unwired: 3 in, 1 out]
            n293 = case shown="True" "Re-save headers" {
              tunnel: w830 -> [_ w846]
              frame False {
                # "Just sit around and feel pretty"
              }
              frame True {
                w854 = ""
                # "Append line of most recent channel names to header file"
                n294 = local read "Channel Names (CAEN)"() -> (w853:string[])
                n295 = local read "Channel Names (9207, ai0:7)"() -> (w861:string[])
                n296 = for {
                  N: w846 -> [_]
                  shift-right: [w885] -> w857
                  shift-left: "" -> [w886]
                  i -> [w890]
                  n297 = Format Into String(initial string="t", w890) -> (resulting string=w888:string)  [unwired: 2 in, 1 out]
                  n298 = Concatenate Strings(w886, w888, "\t") -> (w885:string)
                }
                n299 = for {
                  shift-right: [w883] -> w859
                  shift-left: w854 -> [w884]
                  tunnel: w861 -> [w881] mode=indexing
                  n300 = Concatenate Strings(w884, w881, "\t") -> (w883:string)
                }
                n301 = local read "Channel Names (9207, ai8:15)"() -> (w860:string[])
                n302 = for {
                  tunnel: w853 -> [w875] mode=indexing
                  shift-right: [w873] -> w848
                  shift-left: w854 -> [w872]
                  n303 = Concatenate Strings(w872, w875, " (V)", "\t") -> (w873:string)
                }
                n304 = for {
                  shift-right: [w879] -> w856
                  shift-left: w859 -> [w880]
                  tunnel: w860 -> [w877] mode=indexing
                  n305 = Concatenate Strings(w880, w877, "\t") -> (w879:string)
                }
                n306 = for {
                  tunnel: w853 -> [w870] mode=indexing
                  shift-right: [w868] -> w852
                  shift-left: w848 -> [w867]
                  n307 = Concatenate Strings(w867, w870, " (I)", "\t") -> (w868:string)
                }
                n308 = Get Date/Time String() -> (date string=w865:string)  [unwired: 3 in, 1 out]
                n309 = Format Date/Time String() -> (date/time string=w847:string)  [unwired: 3 in]
                n310 = Build Path(base path=path "D:/Log_data/SC_LOG_HEADERS", name or relative path=w865) -> (appended path=w864:path)
                n311 = Concatenate Strings("Time\t", w857, w856, "Temp A\tTemp B\tHeater Power\tSetpoint\t", w852, "Time in seconds\tTime per cycle\t", w847, "\r\n") -> (w849:string)
                n312 = call <vilib>:"Write Spreadsheet String.vi"("append to file? (new file:F)"=TRUE, "spreadsheet string"=w849, "file path (dialog if empty)"=w864) -> ()  [unwired: 7 in, 2 out]
              }
            }
            n313 = Build Path(base path=path "D:/Log_data/SC_LOG", name or relative path=w838) -> (appended path=w837:path)
            n314 = Format Date/Time String() -> (date/time string=w842:string)  [unwired: 3 in]
            n315 = Array To Spreadsheet String(array=w844, 3:"%.3f" ("format string")) -> (spreadsheet string=w840:string)  [unwired: 1 in]
            n316 = Concatenate Strings(w842, "\t", w840) -> (w836:string)
            n317 = call <vilib>:"Write Spreadsheet String.vi"("append to file? (new file:F)"=TRUE, "spreadsheet string"=w836, "file path (dialog if empty)"=w837) -> ()  [unwired: 7 in, 2 out]
          }
          frame #7 {
            # "Status is True if ANY (armed)\ncondition is met"
            # "Detector P. Alert"
            # "Uninteruptable\n Power Supply Alert"
            # "Temp. Warning"
            # "Arms"
            # "Comm. Alert"
            # "Temperature Alert"
            # "Alarm conditions (Temp)"
            # "Check Alarms and Warnings"
            n318 = Index Array(array=w897) -> (element #1=w896:errorcluster, element #2=w895:errorcluster)  [unwired: 2 in]
            n319 = Unbundle By Name(w941) -> ("error out.status"=w923:bool)
            "NI mod 2&3 status" <- w923
            n320 = Unbundle By Name(w953) -> ("error out.status"=w949:bool)
            "NI mod1 (P) status" <- w949
            n321 = Unbundle By Name(w954) -> ("error out.status"=w952:bool)
            "LakeShore status" <- w952
            n322 = Unbundle By Name(w895) -> ("status"=w950:bool)
            "CAEN 2 status" <- w950
            n323 = Unbundle By Name(w896) -> ("status"=w951:bool)
            "CAEN 1 status" <- w951
            n324 = Build Array(w952, w951, w950, w949, w923) -> (w924:bool[])
            n325 = Build Array("LakeShore", "CAEN 1", "CAEN 2", "NI mod 2&3", "NI mod 1") -> (w919:bool[])
            n326 = call "check_ups.vi"() -> ("Error: no voltages read"=w903:bool, "Timestamp last measured"=→"Timestamp last \nmeasured (UPS)":timestamp, "Minimum input voltage measured"=w913:dbl)  [unwired: 8 in, 1 out]
            "Minimum input voltage measured" <- w913
            n327 = property on="Det.P input #" class="DigNum (strict)"() -> ("Value"=w939:i32)  [unwired: 2 in, 2 out]
            n328 = Or Array Elements(Boolean array=w924) -> (logical OR=→"Comm. status":bool)
            n329 = for {
              tunnel: w924 -> [w957] mode=indexing
              tunnel: w919 -> [w956] mode=indexing
              tunnel: [w955] -> w918 mode=indexing
              n330 = And(x=w957, y=w956) -> (x .and. y?=w955:bool)
            }
            n331 = Index Array(array=w940, index=w939) -> (element=w936:dbl)
            n332 = Less?(x=w913, y="UPS Voltage \nLower Threshold") -> (x < y?=w905:bool)
            n333 = Equal?(x=w913, y=-1.0) -> (x = y?=w904:bool)
            n334 = Less?(x=w936, y="Underpressure threshold") -> (x < y?=w934:bool)
            n335 = Build Array(w905, w904, w903) -> (w902:bool[])
            n336 = Or Array Elements(Boolean array=w918) -> (logical OR=w908:bool)
            n337 = Greater?(x=w936, y="Overpressure threshold") -> (0:w935:bool)
            n338 = Or(x=w935, y=w934) -> (x .or. y?=w933:bool)
            "Det. P. warning" <- w933
            n339 = Or Array Elements(Boolean array=w902) -> (logical OR=w901:bool)
            "Warning" <- w901
            n340 = And(x="UPS", y=w901) -> (x .and. y?=w907:bool)
            n341 = And(x=w933, y="Detector Pressure:") -> (x .and. y?=w909:bool)
            n342 = Build Array("T 1", "T 2", "T 3", "T 4", "T 5", "T 6", "T 7", "T 8") -> (w899:bool[])
            n343 = for {
              tunnel: w898 -> [w958] mode=indexing
              tunnel: w899 -> [w961] mode=indexing
              tunnel: [w960] -> w910 mode=indexing
              tunnel: [w959] -> w925 mode=indexing
              n344 = Less?(x=w958, y="Low Temp threshold") -> (x < y?=w963:bool)
              n345 = Greater?(x=w958, y="High Temp threshold") -> (0:w962:bool)
              n346 = Or(x=w963, y=w962) -> (x .or. y?=w959:bool)
              n347 = And(x=w961, y=w959) -> (x .and. y?=w960:bool)
            }
            n348 = Index Array(array=w925) -> (element #1=→"Boolean":bool, element #2=→"Boolean 2":bool, element #3=→"Boolean 3":bool, element #4=→"Boolean 4":bool, element #5=→"Boolean 5":bool, element #6=→"Boolean 6":bool, element #7=→"element":bool, element #8=→"element 2":bool)  [unwired: 8 in]
            n349 = Build Array (concatenate)(w910, w909, w908, w907) -> (w906:bool[])
            n350 = Or Array Elements(Boolean array=w906) -> (logical OR=w900:bool)
            "Alarm state" <- w900
          }
          frame #8 {
            # "Testing alarm will not interfere"
            # "Act on alarm"
            n351 = Or(x="Test alarm", y=w972) -> (x .or. y?=w973:bool)
            n352 = case shown="True" w973 {
              tunnel: "Test alarm" -> [_ w980]
              tunnel: w970 -> [_ w988]
              tunnel: w966 -> [_ w987]
              tunnel: w969 -> [w976 w978]
              tunnel: "Alarm\nMaster switch" -> [_ w985]
              tunnel: [w976 w979] -> w967
              frame False {
                # "Timer stays at previous value"
              }
              frame True {
                n353 = Get Date/Time In Seconds() -> (seconds since 1Jan1904=w992:timestamp)
                n354 = case shown="True" "\"Sound\" alarm" {
                  frame False {
                  }
                  frame True {
                    n355 = call <vilib>:"Beep.vi"("use system alert? (T)"=FALSE, "duration (msec)"=u32 1000, "frequency (Hz)"="Sound alarm\nFrequency (Hz)") -> ()  [unwired: 9 in]
                  }
                }
                n356 = To Double Precision Float(number=w992) -> (double precision float=w989:dbl)
                n357 = Multiply(x="Repeat Alarm SMS\nevery N minutes", y=60.0) -> (x*y=w981:dbl)
                n358 = Subtract(x=w989, y=w978) -> (x-y=w984:dbl)
                n359 = Greater?(x=w984, y=w981) -> (0:w986:bool)
                n360 = And(x=w985, y=w986) -> (x .and. y?=w983:bool)
                n361 = Or(x=w980, y=w983) -> (x .or. y?=w982:bool)
                n362 = case shown="True" w982 {
                  tunnel: w980 -> [_ w1008]
                  tunnel: w988 -> [_ w1016]
                  tunnel: w987 -> [_ w997]
                  tunnel: [w996 w1006] -> w979
                  tunnel: w978 -> [w996 w1005]
                  frame False {
                    # "Alarm not armed, or defined time has not yet passed"
                  }
                  frame True {
                    # "Average T in Det."
                    n363 = local read "Det.P input #"() -> (w1021:i32)
                    n364 = case shown="True" w1008 {
                      tunnel: ["Error encountered inXAMS! Status:" "TESTING the XAMS alarm. Status:"] -> w1015
                      tunnel: [w1025 w1028] -> w1006
                      tunnel: w1005 -> [_ w1028]
                      frame False {
                        n365 = Get Date/Time In Seconds() -> (seconds since 1Jan1904=w1026:timestamp)
                        n366 = To Double Precision Float(number=w1026) -> (double precision float=w1025:dbl)
                      }
                      frame True {
                      }
                    }
                    n367 = for {
                      tunnel: w997 -> [w1030] mode=indexing
                      tunnel: [w1037] -> w1000 mode=indexing
                      i -> [w1031]
                      n368 = Format Into String(format string="%.0f", w1031) -> (resulting string=w1035:string)  [unwired: 2 in, 1 out]
                      n369 = Format Into String(format string="%.1f", w1030) -> (resulting string=w1033:string)  [unwired: 2 in, 1 out]
                      n370 = Concatenate Strings("\n" ("format string"), w1035, "     " ("format string"), w1033) -> (w1037:string)
                    }
                    n371 = Index Array(array=w1016, index=w1021) -> (element=w1017:dbl)
                    n372 = Array Size(array=w997) -> (size(s)=w1019:i32)
                    n373 = Add Array Elements(numeric array=w997) -> (sum=w1020:dbl)
                    n374 = Format Into String(format string="%.3f", w1017) -> (resulting string=w1011:string)  [unwired: 2 in, 1 out]
                    n375 = Divide(x=w1020, y=w1019) -> (x/y=w1009:dbl)
                    n376 = Format Date/Time String() -> (date/time string=w1013:string)  [unwired: 3 in]
                    n377 = Format Into String(format string="%.2f", w1009) -> (resulting string=w998:string)  [unwired: 2 in, 1 out]
                    n378 = Concatenate Strings(w1015, "\nDate/time: ", w1013, "\nDetector Pressure: ", w1011, " bar", "\nDetector Temperatures (°C):", "\nCh:   Temp:" ("format string"), w1000, "\nAverage detector temperature: ", w998) -> (w1004:string)
                    "Alarm (or test) message" <- w1004
                    n379 = for {
                      tunnel: w1004 -> [w1024]
                      tunnel: "Phone numbers" -> [w1023] mode=indexing
                      n380 = call "send_sms.vi"("Message content"=w1024, "Phone number"=w1023) -> ("standard error"=→"SMS error":string)  [unwired: 8 in, 1 out]
                    }
                  }
                }
              }
            }
            n381 = And(x="Shut off heater \nif Alarm is active", y=w972) -> (x .and. y?=w974:bool)
            "Alarm active 2" <- "Alarm\nMaster switch"
          }
          frame #9 {
            # "Daily e-mail"
            n382 = Get Date/Time In Seconds() -> (seconds since 1Jan1904=w1052:timestamp)
            n383 = To Double Precision Float(number=w1052) -> (double precision float=w1051:dbl)
            n384 = Get Date/Time String(want seconds? (F)=FALSE) -> (time string=w1054:string)  [unwired: 2 in, 1 out]
            n385 = Subtract(x=w1051, y=w1044) -> (x-y=w1050:dbl)
            n386 = Equal?(x=w1054, y="Send status email at time:") -> (x = y?=w1047:bool)
            n387 = Greater?(x=w1050, y=62) -> (0:w1046:bool)
            n388 = Build Array("Send daily email?", w1047, w1046) -> (w1045:bool[])
            n389 = And Array Elements(Boolean array=w1045) -> (logical AND=w1041:bool)
            n390 = Or(x="Send status email now", y=w1041) -> (x .or. y?=w1042:bool)
            n391 = case shown="True" w1042 {
              tunnel: w1039 -> [_ w1059]
              tunnel: w1057 -> [_ w1076]
              tunnel: w1056 -> [_ w1085]
              tunnel: w1044 -> [w1058 _]
              tunnel: [w1058 w1071] -> w1043
              frame False {
              }
              frame True {
                # "Average T in Det."
                n392 = Not Equal To 0?(x="Number of Bonus lines") -> (x != 0?=w1064:bool)
                n393 = case shown="True" w1064 {
                  tunnel: [w1096 w1099] -> w1065
                  tunnel: "Number of Bonus lines" -> [_ w1102]
                  frame False {
                    n394 = Build Array("\n[Flavor text module inactive]") -> (w1096:string[])
                  }
                  frame True {
                    n395 = Build Path(base path=path "C:/Users/xams/Desktop/New XAMS Slow Control", name or relative path="cool_beans.txt") -> (appended path=w1103:path)
                    n396 = call-poly <vilib>:"Read Delimited Spreadsheet.vi"("file path (dialog if empty)"=w1103) -> ("all rows"=w1106:string[][])  [unwired: 9 in, 5 out]
                    n397 = Array Size(array=w1106) -> (size(s)=w1108:i32[])
                    n398 = Index Array(array=w1108) -> (element=w1107:i32)  [unwired: 1 in]
                    n399 = for {
                      N: w1102 -> [_]
                      tunnel: w1107 -> [w1113]
                      tunnel: w1106 -> [w1112]
                      tunnel: [w1109] -> w1100 mode=indexing
                      n400 = Random Number (0-1)() -> (number: 0 to 1=w1116:dbl)
                      n401 = Multiply(x=w1113, y=w1116) -> (x*y=w1115:dbl)
                      n402 = Round To Nearest(number=w1115) -> (nearest integer value=w1114:dbl)
                      n403 = Index Array(array=w1112, index (row)=w1114) -> (element=w1110:string[])  [unwired: 1 in]
                      n404 = Concatenate Strings("\n", w1110) -> (w1109:string)
                    }
                    n405 = Concatenate Strings("\n\nCool beans of the day: ", w1100) -> (w1098:string)
                    n406 = Build Array(w1098) -> (w1099:string[])
                  }
                }
                n407 = local read "Det.P input #"() -> (w1086:i32)
                n408 = for {
                  tunnel: [w1125] -> w1078 mode=indexing
                  tunnel: w1059 -> [w1117] mode=indexing
                  i -> [w1118]
                  n409 = Format Into String(format string="%.0f", w1118) -> (resulting string=w1122:string)  [unwired: 2 in, 1 out]
                  n410 = Format Into String(format string="%.2f", w1117) -> (resulting string=w1120:string)  [unwired: 2 in, 1 out]
                  n411 = Concatenate Strings("\nCh: " ("format string"), w1122, ", Temp: " ("format string"), w1120, "°C." ("format string")) -> (w1125:string)
                }
                n412 = Array Size(array=w1059) -> (size(s)=w1094:i32)
                n413 = Add Array Elements(numeric array=w1059) -> (sum=w1095:dbl)
                n414 = Index Array(array=w1085, index=w1086) -> (element=w1083:dbl)
                n415 = Divide(x=w1095, y=w1094) -> (x/y=w1092:dbl)
                n416 = Format Into String(format string="%.3f", w1083) -> (resulting string=w1081:string)  [unwired: 2 in, 1 out]
                n417 = Format Into String(format string="%.2f", w1092) -> (resulting string=w1075:string)  [unwired: 2 in, 1 out]
                n418 = Select(t="ACTIVE!!!!!", s=w1076, f="inactive.") -> (s? t:f=w1088:string)
                n419 = Concatenate Strings("Hello, XAMS teammembers.", "\n\nThe alarm is currently ", w1088, "\n\nThe latest detector pressure is: ", w1081, " bar." ("format string"), "\nTemperatures inside the detector are:", w1078, "\nThe average detector temperature is ", w1075, "°C." ("format string"), "\n\nThank you for doing your best today, once again!\nRegards, SC.", w1065) -> (w1070:string)
                "Status email preview" <- w1070
                n420 = call "custom_email_program.vi"("mail server"="smtp.nikhef.nl", "return address"="return address", "message"=w1070, "subject ([No Subject])"="XAMS daily status email.", "Email Adresses"="Email Addresses") -> ("error out"=w1062:errorcluster)  [unwired: 6 in]
                n421 = Unbundle By Name(w1062) -> ("code"=→"Email error":i32, "source"=→"source":string)
                n422 = Get Date/Time In Seconds() -> (seconds since 1Jan1904=w1072:timestamp)
                n423 = To Double Precision Float(number=w1072) -> (double precision float=w1071:dbl)
              }
            }
          }
        }
        n424 = Decrement(x="Cycles to execute") -> (x-1=w295:dbl)
        n425 = Decrement(x=w295) -> (x-1=w294:dbl)
        n426 = Greater?(x=w278, y=w294) -> ()  [unwired: 1 out]
        n427 = Decrement(x="Clear data every N cycles") -> (x-1=w275:dbl)
        n428 = Greater?(x=w278, y=w275) -> (0:w277:bool)
        n429 = And(x="Auto-clear data?", y=w277) -> (x .and. y?=w280:bool)
        n430 = Or(x=w280, y="Clear data") -> (x .or. y?=w282:bool)
        n431 = case shown="False" w282 {
          tunnel: w293 -> [w321 _]
          tunnel: [w321 dbl[][] []] -> w292
          tunnel: w291 -> [w320 _]
          tunnel: [w320 w327] -> w290
          tunnel: w289 -> [w319 _]
          tunnel: [w319 w327] -> w288
          tunnel: w287 -> [w318 _]
          tunnel: [w318 w325] -> w286
          tunnel: w285 -> [w317 _]
          tunnel: [w317 w323] -> w284
          tunnel: w278 -> [w316 _]
          tunnel: [w316 0] -> w279
          frame False {
          }
          frame True {
            w327 = 0.0
            n432 = Get Date/Time In Seconds() -> (seconds since 1Jan1904=w324:timestamp)
            n433 = To Double Precision Float(number=w324) -> (double precision float=w326:dbl)
            n434 = Build Array(w324) -> (w323:timestamp[])
            n435 = Build Array(w326, w326) -> (w325:dbl[])
          }
        }
        n436 = Or(x=FALSE, y="stop") -> (x .or. y?=w313:bool)
        "Auto-clear" <- "Auto-clear data?"
      }
    }
    frame True {
    }
  }
  n437 = Array Size(array=w30) -> (size(s)=w33:i32)
  n438 = Decrement(x=w33) -> (x-1=w32:i32)
  n439 = Index Array(array=w30, index #1=w32, index #2=1 ("index")) -> (element #1=w31:timestamp, element #2=w16:timestamp)
  n440 = To Double Precision Float(number=w31) -> (double precision float=w29:dbl)
  n441 = To Double Precision Float(number=w16) -> (double precision float=w28:dbl)
  n442 = flat-sequence {
    tunnel: w23 -> [w1170]
    tunnel: w19 -> [w1142]
    tunnel: w18 -> [w1160]
    tunnel: w11 -> [w1149]
    tunnel: w6 -> [w1146]
    tunnel: w1 -> [w1140]
    frame #0 {
      w1166 = u16 2 items=["1"=1, "2"=2] ("Heater Output (1:1)")
      w1167 = u16 0 items=["Off", "Low (On)", "Medium", "High"] ("Range (0:Off)")
      # "The voltages over the components do NOT get reset by these icons,\nonly the communication gets stopped and references closed."
      # "Important icons! Always press STOP button when done \ninstead of force closing, otherwise these don't get executed"
      # "Turn off heater, shutdown COM"
      # "Error Handling and Post-Processing (EHaPP)"
      n443 = Unbundle(w1170) -> ("VISA resource name out"=w1169:refnum<visa-resource-name>, "error out"=w1168:errorcluster)
      n444 = Unbundle(w1160) -> ("task out"=w1158:refnum<k21>, "error out"=w1156:errorcluster)
      n445 = Unbundle(w1149) -> ("task out"=w1153:refnum<k21>, "error out"=w1151:errorcluster)
      n446 = Unbundle(w1146) -> ("task out"=w1145:refnum<k21>, "error out"=w1144:errorcluster)
      n447 = Index Array(array=w1142) -> (element=w1141:T4)  [unwired: 1 in]
      n448 = Index Array(array=w1140) -> (element #1=w1138:errorcluster, element #2=w1137:errorcluster)  [unwired: 2 in]
      n449 = Merge Errors(w1138, w1137) -> (w1136:errorcluster)
      n450 = Unbundle(w1141) -> ("VISA resource name"=w1161:refnum<visa-resource-name>)  [unwired: 2 out]
      n451 = call <vilib>:"DAQmx Stop Task.vi"("task/channels in"=w1158, "error in"=w1156) -> ("task out"=w1157:refnum<k21>, "error out"=w1155:errorcluster)  [unwired: 12 in]
      n452 = call <vilib>:"DAQmx Stop Task.vi"("task/channels in"=w1153, "error in"=w1151) -> ("task out"=w1152:refnum<k21>, "error out"=w1150:errorcluster)  [unwired: 12 in]
      n453 = call <vilib>:"DAQmx Stop Task.vi"("task/channels in"=w1145, "error in"=w1144) -> ("task out"=w1143:refnum<k21>, "error out"=w1147:errorcluster)  [unwired: 12 in]
      n454 = call <instrlib>:"Configure Output Range and Manual Value.vi"("VISA resource name"=w1169, "Heater Output (1:1)"=w1166, "Range (0:Off)"=w1167, "Manual Output (0.00 %)"=0.0, "error in (no error)"=w1168) -> ("VISA resource name out"=w1164:refnum<visa-resource-name>, "error out"=w1163:errorcluster)  [unwired: 9 in]
      n455 = call <instrlib>:"Close.vi"("VISA resource name"=w1161) -> ("error out"=w1139:errorcluster)  [unwired: 10 in]
      n456 = call <instrlib>:"Close.vi"("error in (no error)"=w1163, "VISA resource name"=w1164) -> ("error out"=w1162:errorcluster)  [unwired: 9 in]
      n457 = call <vilib>:"DAQmx Clear Task.vi"("task in"=w1157, "error in"=w1155) -> ("error out"=w1159:errorcluster)  [unwired: 13 in]
      n458 = call <vilib>:"DAQmx Clear Task.vi"("task in"=w1152, "error in"=w1150) -> ("error out"=w1154:errorcluster)  [unwired: 13 in]
      n459 = call <vilib>:"DAQmx Clear Task.vi"("task in"=w1143, "error in"=w1147) -> ("error out"=w1148:errorcluster)  [unwired: 13 in]
      n460 = Merge Errors(w1139, w1136) -> (w1135:errorcluster)
      n461 = call <vilib>:"Simple Error Handler.vi"("error in (no error)"=w1162) -> ()  [unwired: 4 in, 5 out]
      n462 = call <vilib>:"Simple Error Handler.vi"("error in (no error)"=w1159) -> ()  [unwired: 4 in, 5 out]
      n463 = call <vilib>:"Simple Error Handler.vi"("error in (no error)"=w1154) -> ()  [unwired: 4 in, 5 out]
      n464 = call <vilib>:"Simple Error Handler.vi"("error in (no error)"=w1148) -> ()  [unwired: 4 in, 5 out]
      n465 = call <vilib>:"Simple Error Handler.vi"("error in (no error)"=w1135) -> ()  [unwired: 4 in, 5 out]
    }
  }
  n466 = Subtract(x=w29, y=w28) -> ()  [unwired: 1 out]
  "Started up?" <- w27
